vi "MWT NO STIM.vi"() -> ()   [LabVIEW 2015]
uses:
  <vilib>/userdefined/High Color/IMAQdx.ctl
  <vilib>/vision/Image Controls.llb/IMAQ Image.ctl
  <vilib>/DAQmx/write.llb/DAQmx Write (Digital Bool 1Line 1Point).vi
  <vilib>/Utility/config.llb/Read Key (String).vi
  <vilib>/DAQmx/create/channels.llb/DAQmx Create Channel (DO-Digital Output).vi
  <vilib>/DAQmx/miscellaneous.llb/DAQmx Fill In Error Info.vi
  MWT.dll
  <vilib>/vision/driver/NI_Vision_Acquisition_Software.lvlib
  <vilib>/Utility/config.llb/NI_LVConfig.lvlib
panel:
  out "Go":bool
  in  "Turn on external triggering of camera":bool
  in  "User interface display slector":u16(ring)=2 items=["Raw Image", "Memory Image", "Fixed Image", "Nothing"]
  out "Auto-end in (s)":dbl
  out "error out 2":errorcluster
  in  "Minimum time between events(ms)":u32=2000
  in  "custom 1 timing array":dbl[](array[numeric])=[0.0]
  in  "puff timing array":dbl[](array[numeric])=[0.0]
  in  "tap timing array":dbl[](array[numeric])=[0.0]
  in  "custom 2 timing array":dbl[](array[numeric])=[0.0]
  in  "Tap Train Number":i32[][](array[numeric])=[[0, 1]]
  in  "Turn on Background division algorithm":bool
  in  "custom 2 fraction of time between is active":sgl[][](array[numeric])=[[0.0, 0.5]]
  in  "time between custom 2 onset":i32[][](array[numeric])=[[0, 50]]
  in  "custom 1 fraction of time between is active":sgl[][](array[numeric])=[[0.0, 0.5]]
  in  "time between custom 1 onset":i32[][](array[numeric])=[[0, 50]]
  in  "time between puff onset":i32[][](array[numeric])=[[0, 50]]
  in  "puff fraction of time between is active":sgl[][](array[numeric])=[[0.0, 0.5]]
  in  "time between tap onset":i32[][](array[numeric])=[[0, 10]]
  in  "tap fraction of time between is active":sgl[][](array[numeric])=[[0.0, 0.6]]
  in  "Turn on output aggregation?":bool=TRUE
  out "# Custom 2's Delivered":i32
  out "Time until Next Custom 2":dbl
  in  "Custom 2 Signal-high lead up":i32=20
  in  "Custom 2 Signal-high duration":i32=50
  in  "Advanced Custom 2 Settings":bool
  in  "Custom 2 Stimulus Method":u16(ring) items=["Fixed Interval"=0, "Exponential Interval"=2, "Custom"=5]
  in  "Custom 2 Number":i32 caption="# of Puff events"
  in  "Custom 2 Interval":dbl caption="Custom Interval (s)"
  in  "Custom 2 Delay":dbl caption="Puff Onset Delay (s)" format="%#_4g"
  in  "Custom 2":bool
  out "Image Data Input Source":T1(ring)
  in  "Number of Image Adaptation Bands":i32=10
  out "error out":errorcluster
  in  "AVI path":path
  out "Auto-start in (s)":dbl
  in  "Auto-start delay (s)":i32
  in  "Raw Image Save Interval (s)":dbl
  in  "IMAQdx camera interface name":T2="cam0"
  out "Query for Interface?":bool=TRUE
  out "last acquired buffer":i32
  in  "Advanced Settings":bool
  out "# Custom 1's Delivered":i32
  out "Time until Next Custom 1":dbl caption="No Custom 1s"
  in  "Custom 1 Signal-high lead up":i32=20
  in  "Custom 1 Signal-high duration":i32=50
  out "Tracker Handle":i32=1
  out "IMAQ Session":refnum<k11>
  in  "Advanced Custom 1 Settings":bool
  in  "Custom 1 Stimulus Method":u16(ring) items=["Fixed Interval"=0, "Exponential Interval"=2, "Custom"=5]
  in  "Custom 1 Number":i32 caption="# of Puff events"
  in  "Custom 1 Interval":dbl caption="Custom Interval (s)"
  in  "Custom 1 Delay":dbl caption="Puff Onset Delay (s)" format="%#_4g"
  in  "Custom 1":bool
  in  "Image Binning":u16(ring)=1 items=["1"=1, "2"=2, "3"=3, "4"=4]
  in  "Contour?":bool
  in  "AFG resource name":refnum<k15>="COM1"
  out "Proccessing loop stopped?":bool
  in  "Object Border":i32=20
  out "AFG Settings":dbl[][](array[numeric])=[[0.0, 10.0, 1.0]]
  out "AFG instrument handle":refnum<k15> caption="instrument handle out"
  in  "Puff Signal-high lead up":i32=20
  in  "Puff Signal-high duration":i32=50
  in  "Frames of Adaptation":i32=10
  out "# Taps Delivered":i32
  out "# Puffs Delivered":i32
  in  "Skeletonize?":bool
  out "ROI Array":dbl[][](array[numeric])=[[0.0, 0.0, 2350.0, 1726.0, 0.0, 0.0]]
  out "Time until Next Puff":dbl caption="No Puffs"
  out "Seconds into Experiment":dbl
  out "Objects Found":i32
  in  "Bit Depth from Camera?":bool=TRUE
  in  "Image Bit Depth":u32=8
  in  "Advanced Puff Settings":bool
  in  "Graph Input 4":u16(ring)=9 items=["# objects", "# objects persisting", "Persistence", "Speed", "Angular Speed", "Length", "Relative Length", "Width", "Relative Width", "Aspect", "Relative Aspect", "Head Or Tail Angle", "Pixel Count"]
  in  "Graph Input 3":u16(ring)=3 items=["# objects", "# objects persisting", "Persistence", "Speed", "Angular Speed", "Length", "Relative Length", "Width", "Relative Width", "Aspect", "Relative Aspect", "Head Or Tail Angle", "Pixel Count"]
  in  "Graph Input 2":u16(ring)=1 items=["# objects", "# objects persisting", "Persistence", "Speed", "Angular Speed", "Length", "Relative Length", "Width", "Relative Width", "Aspect", "Relative Aspect", "Head Or Tail Angle", "Pixel Count"]
  in  "Graph Input":u16(ring) items=["# objects", "# objects persisting", "Persistence", "Speed", "Angular Speed", "Length", "Relative Length", "Width", "Relative Width", "Aspect", "Relative Aspect", "Head or Tail Angle", "Pixel Count"]
  out "XY Graph 4":cluster{sgl, sgl}[](graph)
  out "XY Graph 3":cluster{sgl, sgl}[](graph)
  out "XY Graph 2":cluster{sgl, sgl}[](graph)
  out "XY Graph":cluster{sgl, sgl}[](graph)
  out "Time until Next Tap":dbl caption="No Taps"
  in  "Puff Stimulus Method":u16(ring) items=["Fixed Interval"=0, "Exponential Interval"=2, "Custom"=5]
  in  "Tap Pulse Active downtime":i32=120
  in  "Tap Pulse Active duration":i32=120
  in  "Tap Signal-high duration":i32=100
  in  "Tap Signal-high lead up":i32=20
  out "seconds per frame":sgl
  out "error count":i32
  out "First-call":bool=TRUE
  in  "Run":bool
  in  "Adaptation Rate":i32=5 step=1
  out "Directory Exists?":bool
  in  "IMAQ Camera Interface Name":string="img0"
  in  "Display/Don't Display":bool=TRUE
  in  "What to display":u16(ring)=2 items=["Raw Image", "Memory Image", "Fixed Image"]
  out "Image":T3(plugin-control)
  in  "Stop":bool=TRUE
  in  "Set New Reference Object":bool
  in  "Clear Reference Object(s)":bool
  in  "Set Region of Interest":bool
  in  "Clear Region of Interest":bool
  in  "Load":bool
  in  "Save":bool
  in  "Advanced Tap Settings":bool
  in  "Tap Stimulus Method":u16(ring) items=["Fixed Interval"=0, "Exponential Interval"=2, "Custom"=5]
  in  "Puff Number":i32 caption="# of Puff events"
  in  "Puff Interval":dbl caption="Puff Interval (s)"
  in  "Puff Delay":dbl caption="Puff Onset Delay (s)"
  in  "Tap Number":i32 caption="# of Tap events" step=1
  in  "Tap Interval":dbl caption="Tap Interval (s)"
  in  "Tap Delay":dbl caption="Tap Onset Delay (s)"
  in  "Puff":bool
  in  "Tap":bool
  in  "Experiment Duration (s)":dbl
  in  "Prefix":string
  in  "Path":path
  in  "Object Size hysteresis (%)":dbl=10.0 min=0.0001 max=100.0
  in  "Minimum Object Size (pixels)":i32=50
  in  "Maximum Object Size (pixels)":i32=6000
  in  "Fill Hysteresis (%)":dbl=50.0 min=0.0001 max=1000.0
  in  "Object Contrast (%)":dbl=10.0 min=0.0001 max=100.0
  in  "Type of object to track":bool
  # "Display"
  # "Do not display"
  # "Multi-Worm Tracker\n(Release -)\n(Without Stimulus)"
  # "Region of Interest"
  # "Reference Object"
  # "Display"
  # "Object Tracker Settings"
  # "Contrast"
  # "Size"
  # "Bright Objects"
  # "Dark Objects"
  # "Data Ouput Settings"
  # "Stimulus Settings"
  # "On"
  # "On"
  # "On"
  # "On"
  # "Off"
  # "Off"
  # "Off"
  # "Off"
  # "Onset delay (s)"
  # "Interval (s)"
  # "Events (#)"
  # "Configuration"
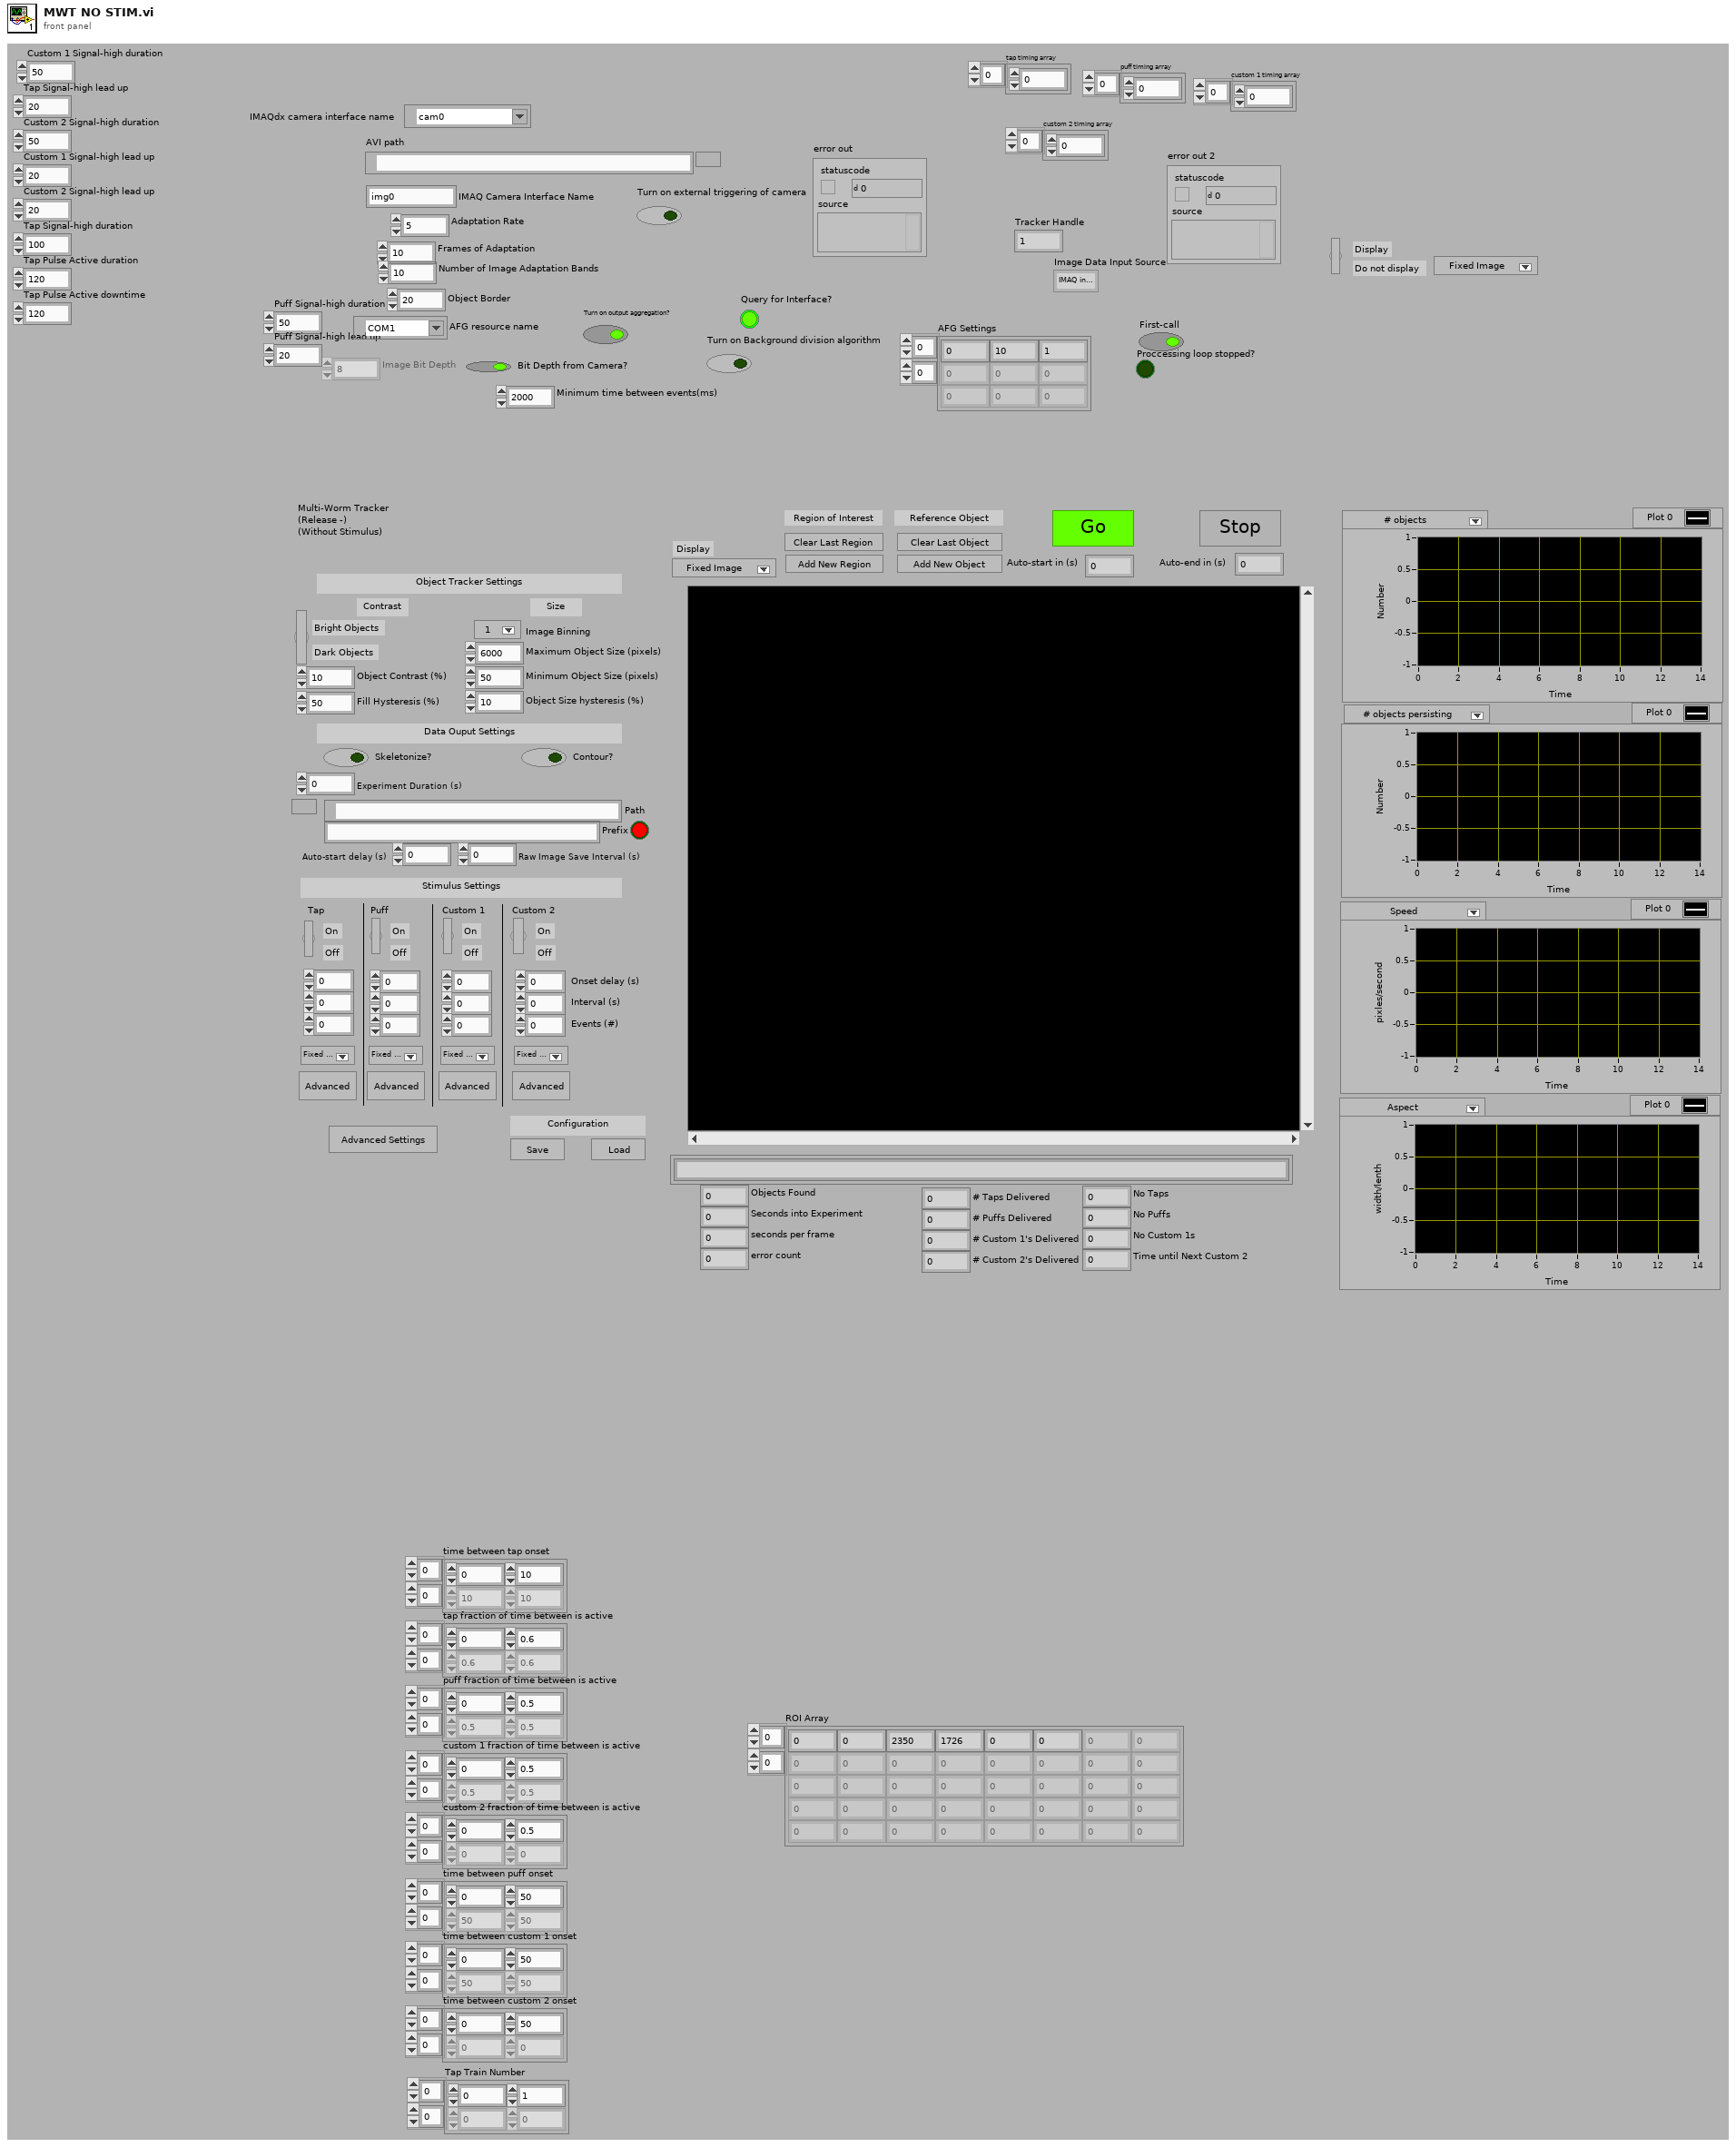
[diagram p1: front panel]
types:
  T1 = enum32{"IMAQ interface", "IMAQdx interface", "AVI file"}
  T2 = typedef "IMAQdx.ctl" = refnum<k21>
  T3 = typedef "IMAQ Image.ctl" = refnum<image>
  T4 = cluster{"Puff":refnum<vi>, "Puff Delay":refnum<vi>, "Puff Interval":refnum<vi>, "Puff Number":refnum<vi>, "Puff Stimulus Method":refnum<vi>}
  T5 = cluster{"Custom 2":refnum<vi>, "Custom 2 Delay":refnum<vi>, "Custom 2 Interval":refnum<vi>, "Custom 2 Number":refnum<vi>, "Custom 2 Stimulus Method":refnum<vi>}
  T6 = cluster{"Custom 1":refnum<vi>, "Custom 1 Delay":refnum<vi>, "Custom 1 Interval":refnum<vi>, "Custom 1 Number":refnum<vi>, "Custom 1 Stimulus Method":refnum<vi>}
  T7 = cluster{"Tap":refnum<vi>, "Tap Delay":refnum<vi>, "Tap Interval":refnum<vi>, "Tap Number":refnum<vi>, "Tap Stimulus Method":refnum<vi>}
  T8 = cluster{cluster{"Tap":refnum<vi>, "Tap Delay":refnum<vi>, "Tap Interval":refnum<vi>, "Tap Number":refnum<vi>, "Tap Stimulus Method":refnum<vi>}, cluster{"Puff":refnum<vi>, "Puff Delay":refnum<vi>, "Puff Interval":refnum<vi>, "Puff Number":refnum<vi>, "Puff Stimulus Method":refnum<vi>}, cluster{"Custom 1":refnum<vi>, "Custom 1 Delay":refnum<vi>, "Custom 1 Interval":refnum<vi>, "Custom 1 Number":refnum<vi>, "Custom 1 Stimulus Method":refnum<vi>}, cluster{"Custom 2":refnum<vi>, "Custom 2 Delay":refnum<vi>, "Custom 2 Interval":refnum<vi>, "Custom 2 Number":refnum<vi>, "Custom 2 Stimulus Method":refnum<vi>}}
  T9 = cluster{"Run":refnum<vi>, "Set Region of Interest":refnum<vi>, "Clear Region of Interest":refnum<vi>, "Clear Reference Object(s)":refnum<vi>, "Set New Reference Object":refnum<vi>, "Advanced Settings":refnum<vi>}
  T10 = cluster{"Path":refnum<vi>, "Prefix":refnum<vi>, "Type of object to track":refnum<vi>, "Object Contrast (%)":refnum<vi>, "Fill Hysteresis (%)":refnum<vi>, "Maximum Object Size (pixels)":refnum<vi>, "Minimum Object Size (pixels)":refnum<vi>, "Object Size hysteresis (%)":refnum<vi>, "Image Binning":refnum<vi>, "Contour?":refnum<vi>, "Skeletonize?":refnum<vi>, "Frames of Adaptation":refnum<vi>, "Adaptation Rate":refnum<vi>, "Object Border":refnum<vi>, "Image Bit Depth":refnum<vi>, "Bit Depth from Camera?":refnum<vi>, "AFG resource name":refnum<vi>, "IMAQ Camera Interface Name":refnum<vi>, "Auto-start delay (s)":refnum<vi>, "Number of Image Adaptation Bands":refnum<vi>, "Experiment Duration (s)":refnum<vi>, "Tap":refnum<vi>, "Tap Delay":refnum<vi>, "Tap Interval":refnum<vi>, "Tap Number":refnum<vi>, "Tap Stimulus Method":refnum<vi>, "Advanced Tap Settings":refnum<vi>, "Puff":refnum<vi>, "Puff Delay":refnum<vi>, "Puff Interval":refnum<vi>, "Puff Number":refnum<vi>, "Puff Stimulus Method":refnum<vi>, "Advanced Puff Settings":refnum<vi>, "Custom 1":refnum<vi>, "Custom 1 Delay":refnum<vi>, "Custom 1 Interval":refnum<vi>, "Custom 1 Number":refnum<vi>, "Custom 1 Stimulus Method":refnum<vi>, "Advanced Custom 1 Settings":refnum<vi>, "puff fraction of time between is active":refnum<vi>, "time between puff onset":refnum<vi>, "tap fraction of time between is active":refnum<vi>, "time between tap onset":refnum<vi>, "Tap Train Number":refnum<vi>, "custom 1 fraction of time between is active":refnum<vi>, "time between custom 1 onset":refnum<vi>, "Custom 2":refnum<vi>, "Custom 2 Delay":refnum<vi>, "Custom 2 Interval":refnum<vi>, "Custom 2 Number":refnum<vi>, "Custom 2 Stimulus Method":refnum<vi>, "Advanced Custom 2 Settings":refnum<vi>, "custom 2 fraction of time between is active":refnum<vi>, "time between custom 2 onset":refnum<vi>, "Save":refnum<vi>, "Load":refnum<vi>, "Raw Image Save Interval (s)":refnum<vi>, "Turn on output aggregation?":refnum<vi>, "Turn on Background division algorithm":refnum<vi>, "Turn on external triggering of camera":refnum<vi>}
  T11 = cluster{cluster{cluster{"Tap":refnum<vi>, "Tap Delay":refnum<vi>, "Tap Interval":refnum<vi>, "Tap Number":refnum<vi>, "Tap Stimulus Method":refnum<vi>}, cluster{"Puff":refnum<vi>, "Puff Delay":refnum<vi>, "Puff Interval":refnum<vi>, "Puff Number":refnum<vi>, "Puff Stimulus Method":refnum<vi>}, cluster{"Custom 1":refnum<vi>, "Custom 1 Delay":refnum<vi>, "Custom 1 Interval":refnum<vi>, "Custom 1 Number":refnum<vi>, "Custom 1 Stimulus Method":refnum<vi>}, cluster{"Custom 2":refnum<vi>, "Custom 2 Delay":refnum<vi>, "Custom 2 Interval":refnum<vi>, "Custom 2 Number":refnum<vi>, "Custom 2 Stimulus Method":refnum<vi>}}, cluster{"Path":refnum<vi>, "Prefix":refnum<vi>, "Type of object to track":refnum<vi>, "Object Contrast (%)":refnum<vi>, "Fill Hysteresis (%)":refnum<vi>, "Maximum Object Size (pixels)":refnum<vi>, "Minimum Object Size (pixels)":refnum<vi>, "Object Size hysteresis (%)":refnum<vi>, "Image Binning":refnum<vi>, "Contour?":refnum<vi>, "Skeletonize?":refnum<vi>, "Frames of Adaptation":refnum<vi>, "Adaptation Rate":refnum<vi>, "Object Border":refnum<vi>, "Image Bit Depth":refnum<vi>, "Bit Depth from Camera?":refnum<vi>, "AFG resource name":refnum<vi>, "IMAQ Camera Interface Name":refnum<vi>, "Auto-start delay (s)":refnum<vi>, "Number of Image Adaptation Bands":refnum<vi>, "Experiment Duration (s)":refnum<vi>, "Tap":refnum<vi>, "Tap Delay":refnum<vi>, "Tap Interval":refnum<vi>, "Tap Number":refnum<vi>, "Tap Stimulus Method":refnum<vi>, "Advanced Tap Settings":refnum<vi>, "Puff":refnum<vi>, "Puff Delay":refnum<vi>, "Puff Interval":refnum<vi>, "Puff Number":refnum<vi>, "Puff Stimulus Method":refnum<vi>, "Advanced Puff Settings":refnum<vi>, "Custom 1":refnum<vi>, "Custom 1 Delay":refnum<vi>, "Custom 1 Interval":refnum<vi>, "Custom 1 Number":refnum<vi>, "Custom 1 Stimulus Method":refnum<vi>, "Advanced Custom 1 Settings":refnum<vi>, "puff fraction of time between is active":refnum<vi>, "time between puff onset":refnum<vi>, "tap fraction of time between is active":refnum<vi>, "time between tap onset":refnum<vi>, "Tap Train Number":refnum<vi>, "custom 1 fraction of time between is active":refnum<vi>, "time between custom 1 onset":refnum<vi>, "Custom 2":refnum<vi>, "Custom 2 Delay":refnum<vi>, "Custom 2 Interval":refnum<vi>, "Custom 2 Number":refnum<vi>, "Custom 2 Stimulus Method":refnum<vi>, "Advanced Custom 2 Settings":refnum<vi>, "custom 2 fraction of time between is active":refnum<vi>, "time between custom 2 onset":refnum<vi>, "Save":refnum<vi>, "Load":refnum<vi>, "Raw Image Save Interval (s)":refnum<vi>, "Turn on output aggregation?":refnum<vi>, "Turn on Background division algorithm":refnum<vi>, "Turn on external triggering of camera":refnum<vi>}, cluster{"Run":refnum<vi>, "Set Region of Interest":refnum<vi>, "Clear Region of Interest":refnum<vi>, "Clear Reference Object(s)":refnum<vi>, "Set New Reference Object":refnum<vi>, "Advanced Settings":refnum<vi>}}
  T12 = cluster{"Value":bool, "Value":dbl, "Value":dbl, "Value":i32, "Value":u16}
  T13 = typedef "AviRefnum.ctl" = refnum<k1>
  T14 = cluster{"IMAQ Session Out":refnum<k11>, "Avi Refnum":T13, "Value":enum32{"IMAQ interface", "IMAQdx interface", "AVI file"}, "Session Out":T2, "Value":bool}
  T15 = cluster{"Value":refnum<k11>, "Value":refnum<k1>, "Value":enum32{"IMAQ interface", "IMAQdx interface", "AVI file"}, cluster{"Value":string, "Value":T2, "Value":path}, bool, "Value":bool}
  T16 = cluster{"Value":string, "Value":T2, "Value":path}
  T17 = cluster{"Value":refnum<k11>, "Value":refnum<k1>, "Value":enum32{"IMAQ interface", "IMAQdx interface", "AVI file"}}
  T18 = cluster{"Value":refnum<k11>, "Value":refnum<k1>, "Value":enum32{"IMAQ interface", "IMAQdx interface", "AVI file"}, "Value":T2, "Value":bool}
  T19 = typedef "Image Type" = u32
  T20 = cluster{"Value":path, "Value":string, "Value":bool, "Value":dbl, "Value":dbl, "Value":i32, "Value":i32, "Value":dbl, "Value":u16, "Value":bool, "Value":bool, "Value":i32, "Value":i32, "Value":i32, "Value":u32, "Value":i32, "Value":bool}
  T21 = cluster{"AFG Settings":dbl[][], "tap timing array":dbl[], "puff timing array":dbl[], "custom timing array":dbl[], "custom 2 timing array":dbl[], cluster{cluster{"Tap":refnum<vi>, "Tap Delay":refnum<vi>, "Tap Interval":refnum<vi>, "Tap Number":refnum<vi>, "Tap Stimulus Method":refnum<vi>}, cluster{"Puff":refnum<vi>, "Puff Delay":refnum<vi>, "Puff Interval":refnum<vi>, "Puff Number":refnum<vi>, "Puff Stimulus Method":refnum<vi>}, cluster{"Custom 1":refnum<vi>, "Custom 1 Delay":refnum<vi>, "Custom 1 Interval":refnum<vi>, "Custom 1 Number":refnum<vi>, "Custom 1 Stimulus Method":refnum<vi>}, cluster{"Custom 2":refnum<vi>, "Custom 2 Delay":refnum<vi>, "Custom 2 Interval":refnum<vi>, "Custom 2 Number":refnum<vi>, "Custom 2 Stimulus Method":refnum<vi>}}, cluster{"Path":refnum<vi>, "Prefix":refnum<vi>, "Type of object to track":refnum<vi>, "Object Contrast (%)":refnum<vi>, "Fill Hysteresis (%)":refnum<vi>, "Maximum Object Size (pixels)":refnum<vi>, "Minimum Object Size (pixels)":refnum<vi>, "Object Size hysteresis (%)":refnum<vi>, "Image Binning":refnum<vi>, "Contour?":refnum<vi>, "Skeletonize?":refnum<vi>, "Frames of Adaptation":refnum<vi>, "Adaptation Rate":refnum<vi>, "Object Border":refnum<vi>, "Image Bit Depth":refnum<vi>, "Bit Depth from Camera?":refnum<vi>, "AFG resource name":refnum<vi>, "IMAQ Camera Interface Name":refnum<vi>, "Auto-start delay (s)":refnum<vi>, "Number of Image Adaptation Bands":refnum<vi>, "Experiment Duration (s)":refnum<vi>, "Tap":refnum<vi>, "Tap Delay":refnum<vi>, "Tap Interval":refnum<vi>, "Tap Number":refnum<vi>, "Tap Stimulus Method":refnum<vi>, "Advanced Tap Settings":refnum<vi>, "Puff":refnum<vi>, "Puff Delay":refnum<vi>, "Puff Interval":refnum<vi>, "Puff Number":refnum<vi>, "Puff Stimulus Method":refnum<vi>, "Advanced Puff Settings":refnum<vi>, "Custom 1":refnum<vi>, "Custom 1 Delay":refnum<vi>, "Custom 1 Interval":refnum<vi>, "Custom 1 Number":refnum<vi>, "Custom 1 Stimulus Method":refnum<vi>, "Advanced Custom 1 Settings":refnum<vi>, "puff fraction of time between is active":refnum<vi>, "time between puff onset":refnum<vi>, "tap fraction of time between is active":refnum<vi>, "time between tap onset":refnum<vi>, "Tap Train Number":refnum<vi>, "custom 1 fraction of time between is active":refnum<vi>, "time between custom 1 onset":refnum<vi>, "Custom 2":refnum<vi>, "Custom 2 Delay":refnum<vi>, "Custom 2 Interval":refnum<vi>, "Custom 2 Number":refnum<vi>, "Custom 2 Stimulus Method":refnum<vi>, "Advanced Custom 2 Settings":refnum<vi>, "custom 2 fraction of time between is active":refnum<vi>, "time between custom 2 onset":refnum<vi>, "Save":refnum<vi>, "Load":refnum<vi>, "Raw Image Save Interval (s)":refnum<vi>, "Turn on output aggregation?":refnum<vi>, "Turn on Background division algorithm":refnum<vi>, "Turn on external triggering of camera":refnum<vi>}, "output values cluster":cluster{"Value":bool, "Value":dbl, "Value":dbl, "Value":dbl, "Value":u16}, "output values cluster":cluster{"Value":bool, "Value":dbl, "Value":dbl, "Value":dbl, "Value":u16}, "output values cluster":cluster{"Value":bool, "Value":dbl, "Value":dbl, "Value":dbl, "Value":u16}, "output values cluster":cluster{"Value":bool, "Value":dbl, "Value":dbl, "Value":dbl, "Value":u16}}
  T22 = cluster{cluster{"Value":refnum<k11>, "Avi Refnum":T13, "Value":enum32{"IMAQ interface", "IMAQdx interface", "AVI file"}, "Value":T2, "Value":bool}, "Value":i32, "Value":i32}
  T23 = cluster{"output values cluster":cluster{"Value":bool, "Value":dbl, "Value":dbl, "Value":dbl, "Value":u16}, "Output Array":dbl[], "output values cluster":cluster{"Value":bool, "Value":dbl, "Value":dbl, "Value":dbl, "Value":u16}, "Output Array":dbl[], "output values cluster":cluster{"Value":bool, "Value":dbl, "Value":dbl, "Value":dbl, "Value":u16}, "Output Array":dbl[], "AFG Settings":dbl[][], "output values cluster":cluster{"Value":bool, "Value":dbl, "Value":dbl, "Value":dbl, "Value":u16}, "Output Array":dbl[]}
  T24 = cluster{cluster{cluster{"Value":refnum<k11>, "Avi Refnum":T13, "Value":enum32{"IMAQ interface", "IMAQdx interface", "AVI file"}, "Value":T2, "Value":bool}, "Value":i32, "Value":i32}, cluster{"Run":refnum<vi>, "Set Region of Interest":refnum<vi>, "Clear Region of Interest":refnum<vi>, "Clear Reference Object(s)":refnum<vi>, "Set New Reference Object":refnum<vi>, "Advanced Settings":refnum<vi>}, "Image Bit Depth":u32}
  T25 = cluster{"Value":bool, "Value":dbl, "Value":dbl, "Value":dbl, "Value":u16}
  T26 = cluster{cluster{cluster{"Value":refnum<k11>, "Avi Refnum":T13, "Value":enum32{"IMAQ interface", "IMAQdx interface", "AVI file"}, "Value":T2, "Value":bool}, "Value":i32, "Value":i32}, cluster{"Path":refnum<vi>, "Prefix":refnum<vi>, "Type of object to track":refnum<vi>, "Object Contrast (%)":refnum<vi>, "Fill Hysteresis (%)":refnum<vi>, "Maximum Object Size (pixels)":refnum<vi>, "Minimum Object Size (pixels)":refnum<vi>, "Object Size hysteresis (%)":refnum<vi>, "Image Binning":refnum<vi>, "Contour?":refnum<vi>, "Skeletonize?":refnum<vi>, "Frames of Adaptation":refnum<vi>, "Adaptation Rate":refnum<vi>, "Object Border":refnum<vi>, "Image Bit Depth":refnum<vi>, "Bit Depth from Camera?":refnum<vi>, "AFG resource name":refnum<vi>, "IMAQ Camera Interface Name":refnum<vi>, "Auto-start delay (s)":refnum<vi>, "Number of Image Adaptation Bands":refnum<vi>, "Experiment Duration (s)":refnum<vi>, "Tap":refnum<vi>, "Tap Delay":refnum<vi>, "Tap Interval":refnum<vi>, "Tap Number":refnum<vi>, "Tap Stimulus Method":refnum<vi>, "Advanced Tap Settings":refnum<vi>, "Puff":refnum<vi>, "Puff Delay":refnum<vi>, "Puff Interval":refnum<vi>, "Puff Number":refnum<vi>, "Puff Stimulus Method":refnum<vi>, "Advanced Puff Settings":refnum<vi>, "Custom 1":refnum<vi>, "Custom 1 Delay":refnum<vi>, "Custom 1 Interval":refnum<vi>, "Custom 1 Number":refnum<vi>, "Custom 1 Stimulus Method":refnum<vi>, "Advanced Custom 1 Settings":refnum<vi>, "puff fraction of time between is active":refnum<vi>, "time between puff onset":refnum<vi>, "tap fraction of time between is active":refnum<vi>, "time between tap onset":refnum<vi>, "Tap Train Number":refnum<vi>, "custom 1 fraction of time between is active":refnum<vi>, "time between custom 1 onset":refnum<vi>, "Custom 2":refnum<vi>, "Custom 2 Delay":refnum<vi>, "Custom 2 Interval":refnum<vi>, "Custom 2 Number":refnum<vi>, "Custom 2 Stimulus Method":refnum<vi>, "Advanced Custom 2 Settings":refnum<vi>, "custom 2 fraction of time between is active":refnum<vi>, "time between custom 2 onset":refnum<vi>, "Save":refnum<vi>, "Load":refnum<vi>, "Raw Image Save Interval (s)":refnum<vi>, "Turn on output aggregation?":refnum<vi>, "Turn on Background division algorithm":refnum<vi>, "Turn on external triggering of camera":refnum<vi>}, "ROI Array":dbl[][], "settings value cluster":cluster{"Value":path, "Value":string, "Value":bool, "Value":dbl, "Value":dbl, "Value":i32, "Value":i32, "Value":dbl, "Value":u16, "Value":bool, "Value":bool, "Value":i32, "Value":i32, "Value":i32, "Value":u32, "Value":i32, "Value":bool}, "AFG Settings":dbl[][], "Output Array":dbl[], "Output Array":dbl[], "Output Array":dbl[], "Output Array":dbl[]}
  T27 = cluster{"Output  ROI Array":dbl[][], "settings value cluster":cluster{"Value":path, "Value":string, "Value":bool, "Value":dbl, "Value":dbl, "Value":i32, "Value":i32, "Value":dbl, "Value":u16, "Value":bool, "Value":bool, "Value":i32, "Value":i32, "Value":i32, "Value":u32, "Value":i32, "Value":bool}, "AFG Settings":dbl[][], "tap timing array":dbl[], "puff timing array":dbl[], "custom timing array":dbl[], "custom 2 timing array":dbl[]}
  T28 = cluster{cluster{"Path":refnum<vi>, "Prefix":refnum<vi>, "Type of object to track":refnum<vi>, "Object Contrast (%)":refnum<vi>, "Fill Hysteresis (%)":refnum<vi>, "Maximum Object Size (pixels)":refnum<vi>, "Minimum Object Size (pixels)":refnum<vi>, "Object Size hysteresis (%)":refnum<vi>, "Image Binning":refnum<vi>, "Contour?":refnum<vi>, "Skeletonize?":refnum<vi>, "Frames of Adaptation":refnum<vi>, "Adaptation Rate":refnum<vi>, "Object Border":refnum<vi>, "Image Bit Depth":refnum<vi>, "Bit Depth from Camera?":refnum<vi>, "AFG resource name":refnum<vi>, "IMAQ Camera Interface Name":refnum<vi>, "Auto-start delay (s)":refnum<vi>, "Number of Image Adaptation Bands":refnum<vi>, "Experiment Duration (s)":refnum<vi>, "Tap":refnum<vi>, "Tap Delay":refnum<vi>, "Tap Interval":refnum<vi>, "Tap Number":refnum<vi>, "Tap Stimulus Method":refnum<vi>, "Advanced Tap Settings":refnum<vi>, "Puff":refnum<vi>, "Puff Delay":refnum<vi>, "Puff Interval":refnum<vi>, "Puff Number":refnum<vi>, "Puff Stimulus Method":refnum<vi>, "Advanced Puff Settings":refnum<vi>, "Custom 1":refnum<vi>, "Custom 1 Delay":refnum<vi>, "Custom 1 Interval":refnum<vi>, "Custom 1 Number":refnum<vi>, "Custom 1 Stimulus Method":refnum<vi>, "Advanced Custom 1 Settings":refnum<vi>, "puff fraction of time between is active":refnum<vi>, "time between puff onset":refnum<vi>, "tap fraction of time between is active":refnum<vi>, "time between tap onset":refnum<vi>, "Tap Train Number":refnum<vi>, "custom 1 fraction of time between is active":refnum<vi>, "time between custom 1 onset":refnum<vi>, "Custom 2":refnum<vi>, "Custom 2 Delay":refnum<vi>, "Custom 2 Interval":refnum<vi>, "Custom 2 Number":refnum<vi>, "Custom 2 Stimulus Method":refnum<vi>, "Advanced Custom 2 Settings":refnum<vi>, "custom 2 fraction of time between is active":refnum<vi>, "time between custom 2 onset":refnum<vi>, "Save":refnum<vi>, "Load":refnum<vi>, "Raw Image Save Interval (s)":refnum<vi>, "Turn on output aggregation?":refnum<vi>, "Turn on Background division algorithm":refnum<vi>, "Turn on external triggering of camera":refnum<vi>}, cluster{"Value":refnum<k11>, "Avi Refnum":T13, "Value":enum32{"IMAQ interface", "IMAQdx interface", "AVI file"}, "Value":T2, "Value":bool}}
  T29 = cluster{cluster{cluster{"Value":refnum<k11>, "Avi Refnum":T13, "Value":enum32{"IMAQ interface", "IMAQdx interface", "AVI file"}, "Value":T2, "Value":bool}, "Value":i32, "Value":i32}, "Image Binning":u16, "Value":u16}
  T30 = cluster{"Acquired Buffer Number":i32, "return type":i32, "destination":i16[][]}
  T31 = cluster{cluster{cluster{"Value":refnum<k11>, "Avi Refnum":T13, "Value":enum32{"IMAQ interface", "IMAQdx interface", "AVI file"}, "Value":T2, "Value":bool}, "Value":i32, "Value":i32}, "ROI Array":dbl[][], "Value":bool, cluster{"Path":refnum<vi>, "Prefix":refnum<vi>, "Type of object to track":refnum<vi>, "Object Contrast (%)":refnum<vi>, "Fill Hysteresis (%)":refnum<vi>, "Maximum Object Size (pixels)":refnum<vi>, "Minimum Object Size (pixels)":refnum<vi>, "Object Size hysteresis (%)":refnum<vi>, "Image Binning":refnum<vi>, "Contour?":refnum<vi>, "Skeletonize?":refnum<vi>, "Frames of Adaptation":refnum<vi>, "Adaptation Rate":refnum<vi>, "Object Border":refnum<vi>, "Image Bit Depth":refnum<vi>, "Bit Depth from Camera?":refnum<vi>, "AFG resource name":refnum<vi>, "IMAQ Camera Interface Name":refnum<vi>, "Auto-start delay (s)":refnum<vi>, "Number of Image Adaptation Bands":refnum<vi>, "Experiment Duration (s)":refnum<vi>, "Tap":refnum<vi>, "Tap Delay":refnum<vi>, "Tap Interval":refnum<vi>, "Tap Number":refnum<vi>, "Tap Stimulus Method":refnum<vi>, "Advanced Tap Settings":refnum<vi>, "Puff":refnum<vi>, "Puff Delay":refnum<vi>, "Puff Interval":refnum<vi>, "Puff Number":refnum<vi>, "Puff Stimulus Method":refnum<vi>, "Advanced Puff Settings":refnum<vi>, "Custom 1":refnum<vi>, "Custom 1 Delay":refnum<vi>, "Custom 1 Interval":refnum<vi>, "Custom 1 Number":refnum<vi>, "Custom 1 Stimulus Method":refnum<vi>, "Advanced Custom 1 Settings":refnum<vi>, "puff fraction of time between is active":refnum<vi>, "time between puff onset":refnum<vi>, "tap fraction of time between is active":refnum<vi>, "time between tap onset":refnum<vi>, "Tap Train Number":refnum<vi>, "custom 1 fraction of time between is active":refnum<vi>, "time between custom 1 onset":refnum<vi>, "Custom 2":refnum<vi>, "Custom 2 Delay":refnum<vi>, "Custom 2 Interval":refnum<vi>, "Custom 2 Number":refnum<vi>, "Custom 2 Stimulus Method":refnum<vi>, "Advanced Custom 2 Settings":refnum<vi>, "custom 2 fraction of time between is active":refnum<vi>, "time between custom 2 onset":refnum<vi>, "Save":refnum<vi>, "Load":refnum<vi>, "Raw Image Save Interval (s)":refnum<vi>, "Turn on output aggregation?":refnum<vi>, "Turn on Background division algorithm":refnum<vi>, "Turn on external triggering of camera":refnum<vi>}, cluster{"Run":refnum<vi>, "Set Region of Interest":refnum<vi>, "Clear Region of Interest":refnum<vi>, "Clear Reference Object(s)":refnum<vi>, "Set New Reference Object":refnum<vi>, "Advanced Settings":refnum<vi>}, "Directory Exists?":refnum<vi>}
  T32 = cluster{cluster{"Value":refnum<k11>, "Avi Refnum":T13, "Value":enum32{"IMAQ interface", "IMAQdx interface", "AVI file"}, "Value":T2, "Value":bool}, i32}
  T33 = cluster{"tap timing array":dbl[], "puff timing array":dbl[], "custom timing array":dbl[], "custom 2 timing array":dbl[]}
  T34 = cluster{"width":u32, "height":u32, "framesPerSecond":u32, "compressionFilter":string, "hasData":bool}
  T35 = cluster{cluster{"Value":refnum<k11>, "Avi Refnum":T13, "Value":enum32{"IMAQ interface", "IMAQdx interface", "AVI file"}, "Value":T2, "Value":bool}, "Value":i32}
  T36 = cluster{"Value":refnum<k11>, "Avi Refnum":T13, "Value":enum32{"IMAQ interface", "IMAQdx interface", "AVI file"}, "Value":T2, "Value":bool}
  T37 = cluster{cluster{cluster{"Value":refnum<k11>, "Avi Refnum":T13, "Value":enum32{"IMAQ interface", "IMAQdx interface", "AVI file"}, "Value":T2, "Value":bool}, "Value":i32}, "Value":i32, "Value":i32, "Value":u16, "Image":T3}
  T38 = cluster{cluster{"Value":refnum<k11>, "Avi Refnum":T13, "Value":enum32{"IMAQ interface", "IMAQdx interface", "AVI file"}, "Value":T2, "Value":bool}, "Acquired Buffer Number":u32}
  T39 = cluster{cluster{"Path":refnum<vi>, "Prefix":refnum<vi>, "Type of object to track":refnum<vi>, "Object Contrast (%)":refnum<vi>, "Fill Hysteresis (%)":refnum<vi>, "Maximum Object Size (pixels)":refnum<vi>, "Minimum Object Size (pixels)":refnum<vi>, "Object Size hysteresis (%)":refnum<vi>, "Image Binning":refnum<vi>, "Contour?":refnum<vi>, "Skeletonize?":refnum<vi>, "Frames of Adaptation":refnum<vi>, "Adaptation Rate":refnum<vi>, "Object Border":refnum<vi>, "Image Bit Depth":refnum<vi>, "Bit Depth from Camera?":refnum<vi>, "AFG resource name":refnum<vi>, "IMAQ Camera Interface Name":refnum<vi>, "Auto-start delay (s)":refnum<vi>, "Number of Image Adaptation Bands":refnum<vi>, "Experiment Duration (s)":refnum<vi>, "Tap":refnum<vi>, "Tap Delay":refnum<vi>, "Tap Interval":refnum<vi>, "Tap Number":refnum<vi>, "Tap Stimulus Method":refnum<vi>, "Advanced Tap Settings":refnum<vi>, "Puff":refnum<vi>, "Puff Delay":refnum<vi>, "Puff Interval":refnum<vi>, "Puff Number":refnum<vi>, "Puff Stimulus Method":refnum<vi>, "Advanced Puff Settings":refnum<vi>, "Custom 1":refnum<vi>, "Custom 1 Delay":refnum<vi>, "Custom 1 Interval":refnum<vi>, "Custom 1 Number":refnum<vi>, "Custom 1 Stimulus Method":refnum<vi>, "Advanced Custom 1 Settings":refnum<vi>, "puff fraction of time between is active":refnum<vi>, "time between puff onset":refnum<vi>, "tap fraction of time between is active":refnum<vi>, "time between tap onset":refnum<vi>, "Tap Train Number":refnum<vi>, "custom 1 fraction of time between is active":refnum<vi>, "time between custom 1 onset":refnum<vi>, "Custom 2":refnum<vi>, "Custom 2 Delay":refnum<vi>, "Custom 2 Interval":refnum<vi>, "Custom 2 Number":refnum<vi>, "Custom 2 Stimulus Method":refnum<vi>, "Advanced Custom 2 Settings":refnum<vi>, "custom 2 fraction of time between is active":refnum<vi>, "time between custom 2 onset":refnum<vi>, "Save":refnum<vi>, "Load":refnum<vi>, "Raw Image Save Interval (s)":refnum<vi>, "Turn on output aggregation?":refnum<vi>, "Turn on Background division algorithm":refnum<vi>, "Turn on external triggering of camera":refnum<vi>}, "appended path":path, "ROI Array":dbl[][], "AFG Settings":dbl[][], "tap timing array":dbl[], "puff timing array":dbl[], "custom timing array":dbl[], "custom 2 timing array":dbl[]}
  T40 = cluster{cluster{"Value":refnum<k11>, "Avi Refnum":T13, "Value":enum32{"IMAQ interface", "IMAQdx interface", "AVI file"}, "Value":T2, "Value":bool}, "Acquired Buffer Number":i32}
  T41 = cluster{"Graph Input":refnum<vi>, "Graph Input 2":refnum<vi>, "Graph Input 3":refnum<vi>, "Graph Input 4":refnum<vi>, "XY Graph":refnum<vi>, "XY Graph 2":refnum<vi>, "XY Graph 3":refnum<vi>, "XY Graph 4":refnum<vi>}
  T42 = cluster{"Value":sgl[][], "Value":i32[][], "Value":i32[][]}
  T43 = cluster{cluster{sgl, sgl}[], cluster{sgl, sgl}[], cluster{sgl, sgl}[], cluster{sgl, sgl}[], cluster{sgl, sgl}[], cluster{sgl, sgl}[], cluster{sgl, sgl}[], cluster{sgl, sgl}[], cluster{sgl, sgl}[], cluster{sgl, sgl}[], cluster{sgl, sgl}[], cluster{sgl, sgl}[], cluster{sgl, sgl}[]}
  T44 = cluster{"custom timing array":dbl[], i32, i32, "Value":bool, i32, "stimulus settings":cluster{"outy3":sgl, "outy3":i32}}
  T45 = cluster{"custom 2 timing array":dbl[], i32, i32, "Value":bool, i32, "stimulus settings":cluster{"outy3":sgl, "outy3":i32}}
  T46 = cluster{"puff timing array":dbl[], i32, i32, "Value":bool, i32, "stimulus settings":cluster{"outy3":sgl, "outy3":i32}}
  T47 = cluster{"tap timing array":dbl[], i32, i32, "Value":bool, i32, "stimulus settings":cluster{"outy3":sgl, "outy3":i32, "Value":i32}}
  T48 = cluster{u32, "millisecond timer value":u32, "millisecond timer value":u32, "Value":u32}
  T49 = cluster{cluster{u32, "millisecond timer value":u32, "millisecond timer value":u32, "Value":u32}, "Time until Next Tap":refnum<vi>, cluster{"tap timing array":dbl[], i32, i32, "Value":bool, i32, "stimulus settings":cluster{"outy3":sgl, "outy3":i32, "Value":i32}}}
  T50 = cluster{cluster{u32, "millisecond timer value":u32, "millisecond timer value":u32, "Value":u32}, "Time until Next Puff":refnum<vi>, cluster{"puff timing array":dbl[], i32, i32, "Value":bool, i32, "stimulus settings":cluster{"outy3":sgl, "outy3":i32}}}
  T51 = cluster{cluster{u32, "millisecond timer value":u32, "millisecond timer value":u32, "Value":u32}, "Time until Next Custom 1":refnum<vi>, cluster{"custom timing array":dbl[], i32, i32, "Value":bool, i32, "stimulus settings":cluster{"outy3":sgl, "outy3":i32}}}
  T52 = cluster{cluster{u32, "millisecond timer value":u32, "millisecond timer value":u32, "Value":u32}, "Time until Next Custom 2":refnum<vi>, cluster{"custom 2 timing array":dbl[], i32, i32, "Value":bool, i32, "stimulus settings":cluster{"outy3":sgl, "outy3":i32}}}
  T53 = cluster{"millisecond timer value":u32, "millisecond timer value":u32, i32, sgl, "Data Cluster":cluster{cluster{sgl, sgl}[], cluster{sgl, sgl}[], cluster{sgl, sgl}[], cluster{sgl, sgl}[], cluster{sgl, sgl}[], cluster{sgl, sgl}[], cluster{sgl, sgl}[], cluster{sgl, sgl}[], cluster{sgl, sgl}[], cluster{sgl, sgl}[], cluster{sgl, sgl}[], cluster{sgl, sgl}[], cluster{sgl, sgl}[]}, "Value":i32, cluster{"Graph Input":refnum<vi>, "Graph Input 2":refnum<vi>, "Graph Input 3":refnum<vi>, "Graph Input 4":refnum<vi>, "XY Graph":refnum<vi>, "XY Graph 2":refnum<vi>, "XY Graph 3":refnum<vi>, "XY Graph 4":refnum<vi>}}
  T54 = cluster{i32, "Tap Number":i32, "Elapsed Time":i32}
  T55 = cluster{"Elapsed Time":i32, "Data Cluster":cluster{cluster{sgl, sgl}[], cluster{sgl, sgl}[], cluster{sgl, sgl}[], cluster{sgl, sgl}[], cluster{sgl, sgl}[], cluster{sgl, sgl}[], cluster{sgl, sgl}[], cluster{sgl, sgl}[], cluster{sgl, sgl}[], cluster{sgl, sgl}[], cluster{sgl, sgl}[], cluster{sgl, sgl}[], cluster{sgl, sgl}[]}}
  T56 = cluster{i32, "Value":i32, "Value":u16, sgl, "Value":u16, "Value":bool, "Value":u32, "Image Out":T3, "Image Pixels (I16)":i16[][], i32[]}
  T57 = cluster{"return value":i32, "return value":i32, "Image Pixels (I16) out":i16[][], "coordinates":i32[]}
  T58 = typedef "NI_LVConfig.lvlib/Config Data RefNum.ctl" = refnum<k1>
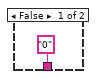
[diagram p2: hidden frame]
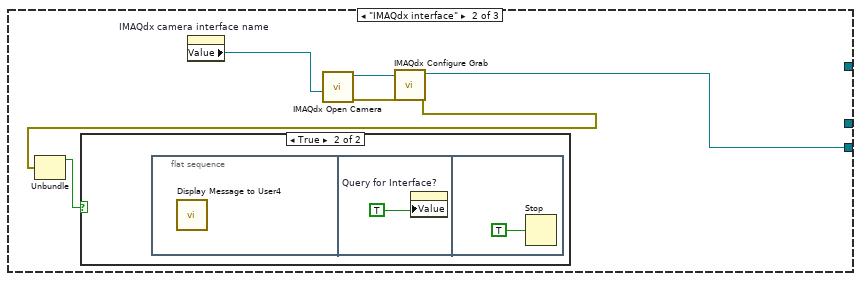
[diagram p5: hidden frame]
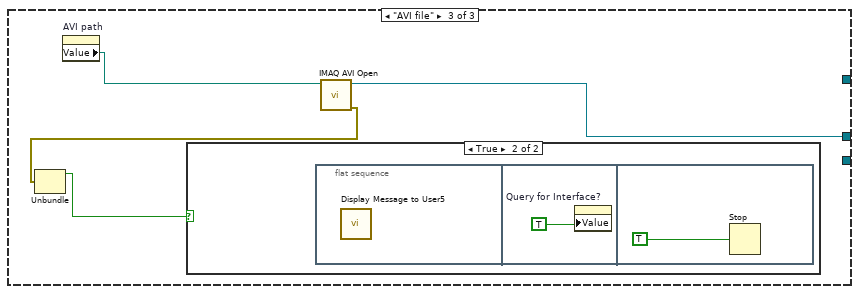
[diagram p7: hidden frame]
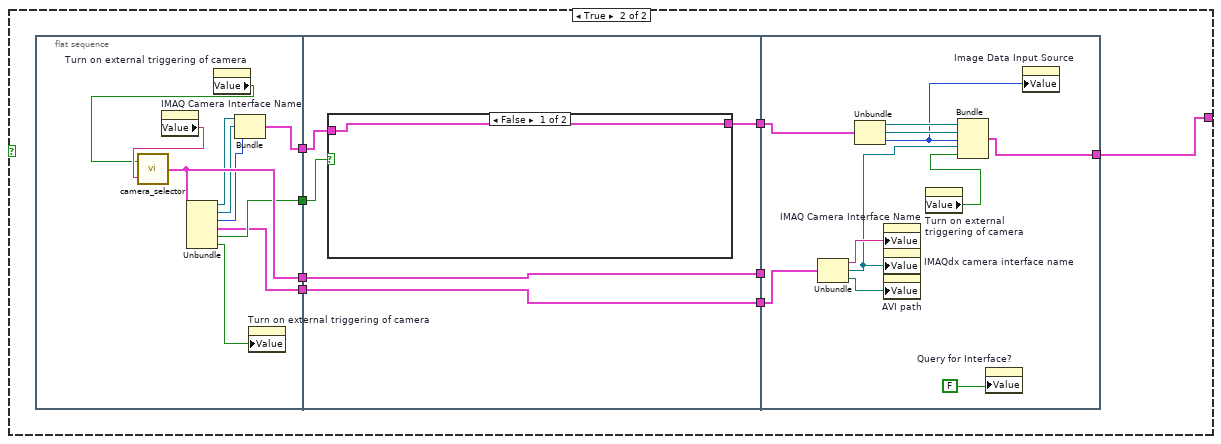
[diagram p9: hidden frame]
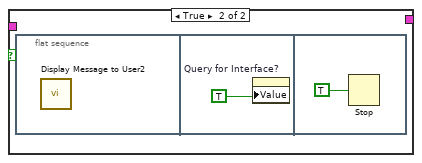
[diagram p10: hidden frame]
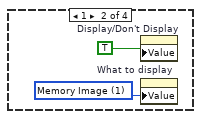
[diagram p16: hidden frame]
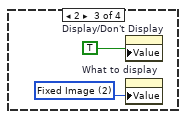
[diagram p17: hidden frame]
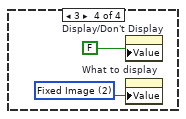
[diagram p18: hidden frame]
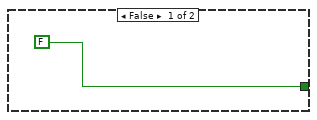
[diagram p19: hidden frame]
diagram:
  w7 = cluster{sgl, sgl}[] [] ("XY Graph")
  w28 = 0
  # "Stimulus counter trigger arrays"
  # "Stimulus event timing arrays"
  # "Copyright (C) 2007 - 2010 Howard Hughes Medical Institute\nCopyright (C) 2007 - 2010 Rex A. Kerr, Nicholas A. Swierczek\n \nThis file is a part of the Multi-Worm Tracker and is distributed under the\nterms of the GNU Lesser General Public Licence version 2.1 (LGPL 2.1).\nFor details, see GPL2.txt and LGPL2.1.txt, or http://www.gnu.org/licences\n \nTo contact the authors, email kerrlab@users.sourceforge.net."
  # "Device Start Timing Control"
  # "Main Controls Cluster"
  # "Assorted buttons for advanced settings/ROI/reference objects"
  # "Stimulus Timing Controls"
  # "Exp. Duration"
  # "Array of ROIs"
  # "Statistics data controls"
  # "Display Controls; \ndisplay type and display on/off toggle"
  # "Settigns-related buttons"
  # "ROI-related buttons"
  # "Reference Object-related buttons"
  # "Overall control buttons"
  # "Image Bit Depth Control"
  # "Function Generator Settings"
  # "Image/Tracking Parameters"
  # "Blob Tracking Parameters"
  # "State variables"
  # "Images"
  # "Hardware System names/handles"
  # "Graph FP objects and controls"
  # "Stimulus delivery control parameters"
  # "Stimulus control signal parameters"
  # "Front panel indicators"
  # "Data output parameters"
  # "References to the front panel controls"
  n1 = control-ref of="AFG resource name"() -> (w74:refnum<vi>)
  n2 = control-ref of="Turn on Background division algorithm"() -> (w8:refnum<vi>)
  n3 = control-ref of="Turn on external triggering of camera"() -> (w6:refnum<vi>)
  n4 = control-ref of="Turn on output aggregation?"() -> (w9:refnum<vi>)
  n5 = control-ref of="Run"() -> (w105:refnum<vi>)
  n6 = control-ref of="Save"() -> (w20:refnum<vi>)
  n7 = control-ref of="Load"() -> (w21:refnum<vi>)
  n8 = control-ref of="Set Region of Interest"() -> (w119:refnum<vi>)
  n9 = control-ref of="Clear Region of Interest"() -> (w122:refnum<vi>)
  n10 = control-ref of="Clear Reference Object(s)"() -> (w121:refnum<vi>)
  n11 = control-ref of="Set New Reference Object"() -> (w120:refnum<vi>)
  n12 = control-ref of="Advanced Settings"() -> (w91:refnum<vi>)
  n13 = control-ref of="Custom 2"() -> (w12:refnum<vi>)
  n14 = control-ref of="Advanced Custom 2 Settings"() -> (w17:refnum<vi>)
  n15 = control-ref of="Tap"() -> (w53:refnum<vi>)
  n16 = control-ref of="Advanced Tap Settings"() -> (w48:refnum<vi>)
  n17 = control-ref of="Puff"() -> (w47:refnum<vi>)
  n18 = control-ref of="Advanced Puff Settings"() -> (w42:refnum<vi>)
  n19 = control-ref of="Custom 1"() -> (w41:refnum<vi>)
  n20 = control-ref of="Advanced Custom 1 Settings"() -> (w36:refnum<vi>)
  n21 = control-ref of="Type of object to track"() -> (w88:refnum<vi>)
  n22 = control-ref of="Contour?"() -> (w81:refnum<vi>)
  n23 = control-ref of="Skeletonize?"() -> (w80:refnum<vi>)
  n24 = control-ref of="Bit Depth from Camera?"() -> (w75:refnum<vi>)
  n25 = control-ref of="Raw Image Save Interval (s)"() -> (w11:refnum<vi>)
  n26 = control-ref of="Custom 2"() -> (w23:refnum<vi>)
  n27 = control-ref of="Custom 2 Delay"() -> (w13:refnum<vi>)
  n28 = control-ref of="Custom 2 Interval"() -> (w14:refnum<vi>)
  n29 = control-ref of="Custom 2 Number"() -> (w15:refnum<vi>)
  n30 = control-ref of="Custom 1"() -> (w96:refnum<vi>)
  n31 = control-ref of="Auto-start delay (s)"() -> (w56:refnum<vi>)
  n32 = control-ref of="Number of Image Adaptation Bands"() -> (w55:refnum<vi>)
  n33 = control-ref of="Experiment Duration (s)"() -> (w54:refnum<vi>)
  n34 = control-ref of="Tap Delay"() -> (w52:refnum<vi>)
  n35 = control-ref of="Tap Interval"() -> (w51:refnum<vi>)
  n36 = control-ref of="Tap Number"() -> (w50:refnum<vi>)
  n37 = control-ref of="Puff Delay"() -> (w46:refnum<vi>)
  n38 = control-ref of="Puff Interval"() -> (w45:refnum<vi>)
  n39 = control-ref of="Puff Number"() -> (w44:refnum<vi>)
  n40 = control-ref of="Custom 1 Delay"() -> (w40:refnum<vi>)
  n41 = control-ref of="Custom 1 Interval"() -> (w39:refnum<vi>)
  n42 = control-ref of="Custom 1 Number"() -> (w38:refnum<vi>)
  n43 = control-ref of="Object Contrast (%)"() -> (w87:refnum<vi>)
  n44 = control-ref of="Fill Hysteresis (%)"() -> (w86:refnum<vi>)
  n45 = control-ref of="Maximum Object Size (pixels)"() -> (w85:refnum<vi>)
  n46 = control-ref of="Minimum Object Size (pixels)"() -> (w84:refnum<vi>)
  n47 = control-ref of="Object Size hysteresis (%)"() -> (w83:refnum<vi>)
  n48 = control-ref of="Frames of Adaptation"() -> (w79:refnum<vi>)
  n49 = control-ref of="Adaptation Rate"() -> (w78:refnum<vi>)
  n50 = control-ref of="Object Border"() -> (w77:refnum<vi>)
  n51 = control-ref of="Image Bit Depth"() -> (w76:refnum<vi>)
  n52 = control-ref of="Puff"() -> (w113:refnum<vi>)
  n53 = control-ref of="custom 2 fraction of time between is active"() -> (w18:refnum<vi>)
  n54 = control-ref of="time between custom 2 onset"() -> (w19:refnum<vi>)
  n55 = control-ref of="Prefix"() -> (w89:refnum<vi>)
  n56 = control-ref of="IMAQ Camera Interface Name"() -> (w73:refnum<vi>)
  n57 = control-ref of="puff fraction of time between is active"() -> (w35:refnum<vi>)
  n58 = control-ref of="time between puff onset"() -> (w34:refnum<vi>)
  n59 = control-ref of="tap fraction of time between is active"() -> (w33:refnum<vi>)
  n60 = control-ref of="time between tap onset"() -> (w32:refnum<vi>)
  n61 = control-ref of="Tap Train Number"() -> (w31:refnum<vi>)
  n62 = control-ref of="custom 1 fraction of time between is active"() -> (w30:refnum<vi>)
  n63 = control-ref of="time between custom 1 onset"() -> (w29:refnum<vi>)
  n64 = control-ref of="Custom 2 Interval"() -> (w25:refnum<vi>)
  n65 = control-ref of="Custom 2 Number"() -> (w26:refnum<vi>)
  n66 = control-ref of="Custom 1 Interval"() -> (w94:refnum<vi>)
  n67 = control-ref of="Custom 1 Number"() -> (w93:refnum<vi>)
  n68 = control-ref of="Custom 2 Delay"() -> (w24:refnum<vi>)
  n69 = control-ref of="Custom 2 Stimulus Method"() -> (w16:refnum<vi>)
  n70 = control-ref of="Tap"() -> (w117:refnum<vi>)
  n71 = control-ref of="Custom 1 Delay"() -> (w95:refnum<vi>)
  n72 = control-ref of="Path"() -> (w90:refnum<vi>)
  n73 = control-ref of="Tap Stimulus Method"() -> (w49:refnum<vi>)
  n74 = control-ref of="Puff Stimulus Method"() -> (w43:refnum<vi>)
  n75 = control-ref of="Custom 1 Stimulus Method"() -> (w37:refnum<vi>)
  n76 = control-ref of="Image Binning"() -> (w82:refnum<vi>)
  n77 = control-ref of="Puff Delay"() -> (w112:refnum<vi>)
  n78 = control-ref of="Puff Interval"() -> (w111:refnum<vi>)
  n79 = control-ref of="Puff Number"() -> (w110:refnum<vi>)
  n80 = control-ref of="Custom 2 Stimulus Method"() -> (w27:refnum<vi>)
  n81 = control-ref of="Tap Delay"() -> (w116:refnum<vi>)
  n82 = control-ref of="Tap Interval"() -> (w115:refnum<vi>)
  n83 = control-ref of="Tap Number"() -> (w114:refnum<vi>)
  n84 = control-ref of="Custom 1 Stimulus Method"() -> (w92:refnum<vi>)
  n85 = control-ref of="Puff Stimulus Method"() -> (w108:refnum<vi>)
  n86 = control-ref of="Tap Stimulus Method"() -> (w109:refnum<vi>)
  n87 = Bundle("Puff"=w113, "Puff Delay"=w112, "Puff Interval"=w111, "Puff Number"=w110, "Puff Stimulus Method"=w108) -> (w106:T4)  [unwired: 1 in]
  n88 = Bundle("Custom 2"=w23, "Custom 2 Delay"=w24, "Custom 2 Interval"=w25, "Custom 2 Number"=w26, "Custom 2 Stimulus Method"=w27) -> (w22:T5)  [unwired: 1 in]
  n89 = Bundle("Custom 1"=w96, "Custom 1 Delay"=w95, "Custom 1 Interval"=w94, "Custom 1 Number"=w93, "Custom 1 Stimulus Method"=w92) -> (w97:T6)  [unwired: 1 in]
  n90 = Bundle("Tap"=w117, "Tap Delay"=w116, "Tap Interval"=w115, "Tap Number"=w114, "Tap Stimulus Method"=w109) -> (w107:T7)  [unwired: 1 in]
  n91 = Bundle(w107, w106, w97, w22) -> (w10:T8)  [unwired: 1 in]
  n92 = Bundle("Run"=w105, "Set Region of Interest"=w119, "Clear Region of Interest"=w122, "Clear Reference Object(s)"=w121, "Set New Reference Object"=w120, "Advanced Settings"=w91) -> (w101:T9)  [unwired: 1 in]
  n93 = Bundle("Path"=w90, "Prefix"=w89, "Type of object to track"=w88, "Object Contrast (%)"=w87, "Fill Hysteresis (%)"=w86, "Maximum Object Size (pixels)"=w85, "Minimum Object Size (pixels)"=w84, "Object Size hysteresis (%)"=w83, "Image Binning"=w82, "Contour?"=w81, "Skeletonize?"=w80, "Frames of Adaptation"=w79, "Adaptation Rate"=w78, "Object Border"=w77, "Image Bit Depth"=w76, "Bit Depth from Camera?"=w75, "AFG resource name"=w74, "IMAQ Camera Interface Name"=w73, "Auto-start delay (s)"=w56, "Number of Image Adaptation Bands"=w55, "Experiment Duration (s)"=w54, "Tap"=w53, "Tap Delay"=w52, "Tap Interval"=w51, "Tap Number"=w50, "Tap Stimulus Method"=w49, "Advanced Tap Settings"=w48, "Puff"=w47, "Puff Delay"=w46, "Puff Interval"=w45, "Puff Number"=w44, "Puff Stimulus Method"=w43, "Advanced Puff Settings"=w42, "Custom 1"=w41, "Custom 1 Delay"=w40, "Custom 1 Interval"=w39, "Custom 1 Number"=w38, "Custom 1 Stimulus Method"=w37, "Advanced Custom 1 Settings"=w36, "puff fraction of time between is active"=w35, "time between puff onset"=w34, "tap fraction of time between is active"=w33, "time between tap onset"=w32, "Tap Train Number"=w31, "custom 1 fraction of time between is active"=w30, "time between custom 1 onset"=w29, "Custom 2"=w12, "Custom 2 Delay"=w13, "Custom 2 Interval"=w14, "Custom 2 Number"=w15, "Custom 2 Stimulus Method"=w16, "Advanced Custom 2 Settings"=w17, "custom 2 fraction of time between is active"=w18, "time between custom 2 onset"=w19, "Save"=w20, "Load"=w21, "Raw Image Save Interval (s)"=w11, "Turn on output aggregation?"=w9, "Turn on Background division algorithm"=w8, "Turn on external triggering of camera"=w6) -> (w102:T10)  [unwired: 1 in]
  n94 = Cluster To Array(cluster=w101) -> (array=w118:refnum<vi>[])
  n95 = call "make_buttons_available.vi"("array"=w118, "Make Available"=TRUE) -> ()
  n96 = call "make_controls_available.vi"("input cluster"=w102, "Make Available"=TRUE) -> ()
  n97 = Bundle(w10, w102, w101) -> (w100:T11)  [unwired: 1 in]
  n98 = flat-sequence {
    tunnel: [w125] -> w68
    tunnel: [w123] -> w67
    tunnel: w100 -> [w125]
    tunnel: [w207] -> w99
    tunnel: w68 -> [w207]
    tunnel: w67 -> [w195]
    tunnel: [w195] -> w66
    tunnel: w99 -> [w224]
    tunnel: [w224] -> w62
    tunnel: [w234] -> w60
    tunnel: w66 -> [w229]
    tunnel: [w228] -> w58
    tunnel: w62 -> [w378]
    tunnel: [w378] -> w61
    tunnel: w60 -> [w377]
    tunnel: [w377] -> w59
    tunnel: w58 -> [w376]
    tunnel: [w376] -> w57
    tunnel: [w373] -> w4
    tunnel: w61 -> [w426]
    tunnel: [w392] -> w98
    tunnel: w59 -> [w392]
    tunnel: [w426] -> w71
    tunnel: w57 -> [w420]
    tunnel: [w415] -> w65
    tunnel: [w399] -> w63
    tunnel: w4 -> [w384]
    tunnel: [w384] -> w3
    tunnel: w98 -> [w506]
    tunnel: [w479] -> w72
    tunnel: w71 -> [w479]
    tunnel: w65 -> [w472]
    tunnel: [w476] -> w64
    tunnel: w63 -> [w475]
    tunnel: w3 -> [w437]
    tunnel: [w437] -> w2
    tunnel: w72 -> [w804]
    tunnel: w64 -> [w802]
    tunnel: w2 -> [w799]
    frame #0 {
      n99 = property on="Query for Interface?" class="Bool (strict)"() -> ("Value"=w124:bool)  [unwired: 2 in, 2 out]
      n100 = case shown="False" w124 {
        tunnel: [w127 w154] -> w123
        frame False {
          n101 = property on="Image Data Input Source" class="Enum (strict)"() -> ("Value"=w129:T1)  [unwired: 2 in, 2 out]
          n102 = case shown="\"IMAQ interface\", Default" w129 {
            tunnel: [_ w141 _] -> w128
            tunnel: [w137 _ _] -> w131
            tunnel: [_ _ w150] -> w130
            frame "IMAQ interface", Default {
              n103 = property on="IMAQ Camera Interface Name" class="Str"() -> ("Value"=w134:string)  [unwired: 2 in, 2 out]
              n104 = call <vilib>:"IMAQ Init.vi"("Interface Name"=w134) -> ("error out"=w136:errorcluster, "IMAQ Session Out"=w135:refnum<k11>)  [unwired: 9 in]
              n105 = call <vilib>:"IMAQ Grab Setup.vi"("error in (no error)"=w136, "IMAQ Session In"=w135) -> ("error out"=w133:errorcluster, "IMAQ Session Out"=w137:refnum<k11>)  [unwired: 8 in]
              n106 = Unbundle(w133) -> ("status"=w132:bool)  [unwired: 2 out]
              n107 = case shown="True" w132 {
                frame False {
                }
                frame True {
                  n108 = flat-sequence {
                    frame #0 {
                      n109 = call "Display Message to User3"() -> ()  [unwired: 10 in, 2 out]
                    }
                    frame #1 {
                      n110 = property on="Query for Interface?" class="Bool (strict)"("Value"=TRUE ("Query for Interface?")) -> ()  [unwired: 2 in, 2 out]
                    }
                    frame #2 {
                      n111 = Stop(stop? (T)=TRUE) -> ()
                    }
                  }
                }
              }
            }
            frame "IMAQdx interface" {
              n112 = property on="IMAQdx camera interface name" class="IMAQdx (strict)"() -> ("Value"=w142:T2)  [unwired: 2 in, 2 out]
              n113 = call <vilib>:"IMAQdx Open Camera.vi"("Session In"=w142) -> ("error out"=w144:errorcluster, "Session Out"=w143:T2)  [unwired: 9 in]
              n114 = call <vilib>:"IMAQdx Configure Grab.vi"("error in"=w144, "Session In"=w143) -> ("error out"=w140:errorcluster, "Session Out"=w141:T2)  [unwired: 8 in]
              n115 = Unbundle(w140) -> ("status"=w145:bool)  [unwired: 2 out]
              n116 = case shown="True" w145 {
                frame False {
                }
                frame True {
                  n117 = flat-sequence {
                    frame #0 {
                      n118 = call "Display Message to User4"() -> ()  [unwired: 10 in, 2 out]
                    }
                    frame #1 {
                      n119 = property on="Query for Interface?" class="Bool (strict)"("Value"=TRUE ("Query for Interface?")) -> ()  [unwired: 2 in, 2 out]
                    }
                    frame #2 {
                      n120 = Stop(stop? (T)=TRUE) -> ()
                    }
                  }
                }
              }
            }
            frame "AVI file" {
              n121 = property on="AVI path" class="Path"() -> ("Value"=w151:path)  [unwired: 2 in, 2 out]
              n122 = call "IMAQ AVI Open"("AVI Path"=w151) -> ("error out"=w148:errorcluster, "Avi Refnum"=w150:T13)  [unwired: 9 in]
              n123 = Unbundle(w148) -> ("status"=w149:bool)  [unwired: 2 out]
              n124 = case shown="True" w149 {
                frame False {
                }
                frame True {
                  n125 = flat-sequence {
                    frame #0 {
                      n126 = call "Display Message to User5"() -> ()  [unwired: 10 in, 2 out]
                    }
                    frame #1 {
                      n127 = property on="Query for Interface?" class="Bool (strict)"("Value"=TRUE ("Query for Interface?")) -> ()  [unwired: 2 in, 2 out]
                    }
                    frame #2 {
                      n128 = Stop(stop? (T)=TRUE) -> ()
                    }
                  }
                }
              }
            }
          }
          n129 = property on="Turn on external triggering of camera" class="Bool (strict)"() -> ("Value"=w126:bool)  [unwired: 2 in, 2 out]
          n130 = Bundle("IMAQ Session Out"=w131, "Avi Refnum"=w130, "Value"=w129, "Session Out"=w128, "Value"=w126) -> (w127:T14)  [unwired: 1 in]
        }
        frame True {
          n131 = flat-sequence {
            tunnel: [w164] -> w161
            tunnel: [w170] -> w159
            tunnel: [w169] -> w157
            tunnel: [w168] -> w156
            tunnel: w161 -> [w176]
            tunnel: [w176] -> w160
            tunnel: w159 -> [w175]
            tunnel: [w175] -> w158
            tunnel: w157 -> [w174]
            tunnel: w156 -> [w173]
            tunnel: [w172] -> w155
            tunnel: w160 -> [w189]
            tunnel: w158 -> [_]
            tunnel: w155 -> [w188]
            tunnel: [w187] -> w154
            frame #0 {
              n132 = property on="IMAQ Camera Interface Name" class="Str"() -> ("Value"=w171:string)  [unwired: 2 in, 2 out]
              n133 = property on="Turn on external triggering of camera" class="Bool (strict)"() -> ("Value"=w162:bool)  [unwired: 2 in, 2 out]
              n134 = call "camera_selector.vi"("IMAQ interface name"=w171, "Use external trigger for camera control (IMAQ only)"=w162) -> ("output cluster"=w170:T15)
              n135 = Unbundle(w170) -> ("Value"=w167:refnum<k11>, "Value"=w166:refnum<k1>, "Value"=w165:T1, w164:T16, w169:bool, "Value"=w163:bool)
              n136 = Bundle("Value"=w167, "Value"=w166, "Value"=w165) -> (w168:T17)  [unwired: 1 in]
              n137 = property on="Turn on external triggering of camera" class="Bool (strict)"("Value"=w163) -> ()  [unwired: 2 in, 2 out]
            }
            frame #1 {
              n138 = case shown="False" w174 {
                tunnel: w173 -> [w177 _]
                tunnel: [w177 _] -> w172
                frame False {
                }
                frame True {
                  n139 = flat-sequence {
                    frame #0 {
                      n140 = call "Display Message to User2"() -> ()  [unwired: 10 in, 2 out]
                    }
                    frame #1 {
                      n141 = property on="Query for Interface?" class="Bool (strict)"("Value"=TRUE ("Query for Interface?")) -> ()  [unwired: 2 in, 2 out]
                    }
                    frame #2 {
                      n142 = Stop(stop? (T)=TRUE) -> ()
                    }
                  }
                }
              }
            }
            frame #2 {
              n143 = Unbundle(w189) -> ("Value"=w190:string, "Value"=w182:T2, "Value"=w181:path)
              n144 = Unbundle(w188) -> ("Value"=w186:refnum<k11>, "Value"=w185:refnum<k1>, "Value"=w183:T1)
              n145 = property on="IMAQ Camera Interface Name" class="Str"("Value"=w190) -> ()  [unwired: 2 in, 2 out]
              n146 = property on="IMAQdx camera interface name" class="IMAQdx (strict)"("Value"=w182) -> ()  [unwired: 2 in, 2 out]
              n147 = property on="AVI path" class="Path"("Value"=w181) -> ()  [unwired: 2 in, 2 out]
              n148 = property on="Turn on external triggering of camera" class="Bool (strict)"() -> ("Value"=w180:bool)  [unwired: 2 in, 2 out]
              n149 = Bundle("Value"=w186, "Value"=w185, "Value"=w183, "Value"=w182, "Value"=w180) -> (w187:T18)  [unwired: 1 in]
              n150 = property on="Query for Interface?" class="Bool (strict)"("Value"=FALSE ("Query for Interface?")) -> ()  [unwired: 2 in, 2 out]
              n151 = property on="Image Data Input Source" class="Enum (strict)"("Value"=w183) -> ()  [unwired: 2 in, 2 out]
            }
          }
        }
      }
    }
    frame #1 {
      w208 = T19 1 items=["Grayscale (U8)", "Grayscale (I16)", "Grayscale (SGL)", "Complex (CSG)", "RGB (U32)", "HSL (U32)", "RGB (U64)"] ("Image Type")
      # "MWT_getNewHandle"
      # "Create memory for displayed image"
      # "Dis/enable run button"
      # "Set initial state of important buttons"
      # "Initial Set up"
      n152 = disable-structure shown="Disabled" {
        frame Disabled {
          # "Stimulus Delivery Setup"
          n153 = call "Init_Stimulus.vi"() -> ()  [unwired: 1 in]
        }
        frame Enabled {
        }
      }
      n154 = property on="Stop" class="Bool (strict)"("Disabled"=u8 0, "Value"=FALSE) -> ()  [unwired: 2 in, 2 out]
      n155 = property on="Run" class="Bool (strict)"("Value"=FALSE) -> ()  [unwired: 2 in, 2 out]
      n156 = property on="Display/Don't Display" class="Bool (strict)"("Value"=TRUE) -> ()  [unwired: 2 in, 2 out]
      n157 = Unbundle(w207) -> (w193:T10)  [unwired: 2 out]
      n158 = property on="last acquired buffer" class="DigNum (strict)"("Value"=0 ("last acquired buffer")) -> ()  [unwired: 2 in, 2 out]
      n159 = local read "ROI Array"() -> (w214:dbl[][])
      n160 = call "init_ROI.vi"("Input ROI Array"=w214, "camera cluster"=w195) -> ("First Call? out"=w212:bool, "Output ROI Array"=w213:dbl[][])
      n161 = dll-call lib="C:/_WORKSPACE/DATA/PROJECTS/IMAQ/SOFTWARE/MWT NO STIM/MWT.dll" fn="MWT_getNewHandle"() -> ("return type"=w192:i32)  [unwired: 3 in, 2 out]
      "Tracker Handle" <- w192
      n162 = local write "First-call"(w212) -> ()
      n163 = call "set_in_library.vi"("Cluster"=w193, "camera cluster"=w195, "Tracker Handle"=w192, "Array"=w213) -> ("Directory Exists?"=w201:bool)  [unwired: 1 out]
      n164 = call "BitsPerPixel.vi"("camera cluster"=w195) -> ("BitsPerPixel"=w198:u32)
      n165 = call "GetWidthAndHeight.vi"("camera cluster"=w195) -> ("Width"=w197:u32, "Height"=w196:u32)
      n166 = local write "ROI Array"(w213) -> ()
      n167 = control-ref of="Directory Exists?"() -> (w200:refnum<vi>)
      n168 = call "IMAQ Create"("Image Name"="image data", "Image Type"=w208) -> ("New Image"=w211:T3, "error out"=w191:errorcluster)  [unwired: 3 in]
      n169 = Greater?(x=w198, y=u32 8) -> (0:w205:bool)
      n170 = Select(t=0, s=w201, f=2) -> (s? t:f=w202:i32)
      n171 = property on="Run" class="Bool (strict)"("Disabled"=w202) -> ()  [unwired: 2 in, 2 out]
      n172 = case shown="True" FALSE {
        tunnel: w205 -> [_ w219]
        frame False {
        }
        frame True {
          n173 = case shown="False" w219 {
            frame False {
              n174 = call "Display Message to User"() -> ()  [unwired: 10 in, 2 out]
            }
            frame True {
              # "Everything\nis fine."
            }
          }
        }
      }
      n175 = property class="Bool (strict)"(reference=w200, "Value"=w201) -> ()  [unwired: 1 in, 2 out]
      n176 = call "IMAQ SetImageSize"("error in (no error)"=w191, "Y Resolution"=w196, "X Resolution"=w197, "Image"=w211) -> ("Image Out"=w210:T3)  [unwired: 1 in, 1 out]
      n177 = property on="Image" class="ImageControl"("Value"=w210) -> ()  [unwired: 2 in, 2 out]
    }
    frame #2 {
      # "Initial feedback and settings configuration"
      # "Initial Constants with dummy values"
      n178 = local read "custom 1 timing array"() -> (w222:dbl[])
      n179 = local read "custom 2 timing array"() -> (w223:dbl[])
      n180 = local read "puff timing array"() -> (w221:dbl[])
      n181 = local read "tap timing array"() -> (w220:dbl[])
      n182 = local read "AFG resource name"() -> (w230:refnum<k15>)
      n183 = Unbundle(w224) -> (w225:T10)  [unwired: 2 out]
      n184 = call "get_tracker_settings.vi"("Cluster"=w225) -> ("settings value cluster"=w237:T20)
      n185 = while {
        shift-right: [w247] -> w235
        shift-left: w220 -> [w308]
        shift-right: [w311] -> _
        shift-left: T12 {"Value"=FALSE, "Value"=-1000.0, "Value"=-1000.0, "Value"=1000, "Value"=1000} ("output values cluster") -> [w280]
        shift-right: [w254] -> _
        shift-left: w237 -> [w314]
        shift-right: [w305] -> _
        shift-left: T12 {"Value"=FALSE, "Value"=-1000.0, "Value"=-1000.0, "Value"=1000, "Value"=1000} ("output values cluster") -> [w279]
        shift-right: [w246] -> w236
        shift-left: w221 -> [w307]
        shift-right: [w317] -> _
        shift-left: w230 -> [w318]
        tunnel: w224 -> [w301]
        shift-right: [w245] -> w232
        shift-left: w222 -> [w306]
        shift-right: [w304] -> _
        shift-left: T12 {"Value"=FALSE, "Value"=-1000.0, "Value"=-1000.0, "Value"=1000, "Value"=1000} ("output values cluster") -> [w278]
        shift-right: [w303] -> _
        shift-left: TRUE -> [w302]
        tunnel: w229 -> [w268]
        tunnel: [w268] -> w228
        shift-right: [w275] -> _
        shift-left: T12 {"Value"=FALSE, "Value"=-1000.0, "Value"=-1000.0, "Value"=1000, "Value"=1000} ("output values cluster") -> [w277]
        shift-right: [w244] -> w226
        shift-left: w223 -> [w276]
        stop <- w286 stop-if-true
        # "Note: Condition necessary\nbecause of potential discrepency\nbetween closing camera sessions\nand exiting the VI."
        # "Logic for \"begin after ... seconds\" function"
        # "Dis/enable run button"
        # "Feedback on setup stage"
        # "UI for ROIs"
        # "UI for advanced settings"
        # "UI for reference objects"
        # "Sets values in library,\nas well as saving and loading"
        # "Sets up the timing arrays \nfor the stimuli"
        # "Clean-up if stop is pressed."
        n186 = disable-structure shown="Disabled" {
          disable-tunnel: w318 -> [w325 _]
          disable-tunnel: [w324 _] -> w317
          disable-tunnel: [w321 _] -> w303
          disable-tunnel: w302 -> [w320 _]
          frame Disabled {
            # "AFG initialization"
            n187 = local read "AFG resource name"() -> (w326:refnum<k15>)
            n188 = Not Equal?(x=w326, y=w325) -> (x != y?=w323:bool)
            n189 = And(x=w323, y=w320) -> (x .and. y?=w322:bool)
            n190 = case shown="True" w322 {
              tunnel: [w328 w331] -> w324
              tunnel: w326 -> [_ w331]
              tunnel: w325 -> [w328 _]
              tunnel: [w327 FALSE] -> w321
              tunnel: w320 -> [w327 _]
              frame False {
              }
              frame True {
                n191 = call "AFG_Init.vi"("amplitude (1)"=1.0, "resource name"=w331, "frequency (1000000)"=100.0) -> ("instrument handle out"=w329:refnum<k15>)
                n192 = local write "AFG instrument handle"(w329) -> ()
              }
            }
          }
          frame Enabled {
          }
        }
        n193 = Unbundle(w301) -> (w281:T8, w270:T10)  [unwired: 1 out]
        n194 = Unbundle(w301) -> (w269:T9)  [unwired: 2 out]
        n195 = property on="User interface display slector" class="Ring (strict)"() -> ("Value"=w243:u16)  [unwired: 2 in, 2 out]
        n196 = case shown="0, Default" w243 {
          frame 0, Default {
            w334 = u16 0 items=["Raw Image", "Memory Image", "Fixed Image"] ("What to display")
            n197 = property on="Display/Don't Display" class="Bool (strict)"("Value"=TRUE ("Display/Don't Display")) -> ()  [unwired: 2 in, 2 out]
            n198 = property on="What to display" class="Ring (strict)"("Value"=w334) -> ()  [unwired: 2 in, 2 out]
          }
          frame 1 {
            w336 = u16 1 items=["Raw Image", "Memory Image", "Fixed Image"] ("What to display")
            n199 = property on="Display/Don't Display" class="Bool (strict)"("Value"=TRUE ("Display/Don't Display")) -> ()  [unwired: 2 in, 2 out]
            n200 = property on="What to display" class="Ring (strict)"("Value"=w336) -> ()  [unwired: 2 in, 2 out]
          }
          frame 2 {
            w338 = u16 2 items=["Raw Image", "Memory Image", "Fixed Image"] ("What to display")
            n201 = property on="Display/Don't Display" class="Bool (strict)"("Value"=TRUE ("Display/Don't Display")) -> ()  [unwired: 2 in, 2 out]
            n202 = property on="What to display" class="Ring (strict)"("Value"=w338) -> ()  [unwired: 2 in, 2 out]
          }
          frame 3 {
            w340 = u16 2 items=["Raw Image", "Memory Image", "Fixed Image"] ("What to display")
            n203 = property on="Display/Don't Display" class="Bool (strict)"("Value"=FALSE ("Display/Don't Display")) -> ()  [unwired: 2 in, 2 out]
            n204 = property on="What to display" class="Ring (strict)"("Value"=w340) -> ()  [unwired: 2 in, 2 out]
          }
        }
        n205 = local read "AFG Settings"() -> (w309:dbl[][])
        n206 = local read "Image Bit Depth"() -> (w264:u32)
        n207 = property on="Tracker Handle" class="DigNum (strict)"() -> ("Value"=w316:i32)  [unwired: 2 in, 2 out]
        n208 = property on="last acquired buffer" class="DigNum (strict)"() -> ("Value"=w292:i32)  [unwired: 2 in, 2 out]
        n209 = Bundle("AFG Settings"=w309, "tap timing array"=w308, "puff timing array"=w307, "custom timing array"=w306, "custom 2 timing array"=w276, w281, w270, "output values cluster"=w280, "output values cluster"=w279, "output values cluster"=w278, "output values cluster"=w277) -> (w310:T21)  [unwired: 1 in]
        n210 = Bundle(w268, "Value"=w316, "Value"=w292) -> (w313:T22)  [unwired: 1 in]
        n211 = call "all_things_stimulus.vi"("input cluster"=w310) -> ("output cluster"=w312:T23)
        n212 = Bundle(w313, w269, "Image Bit Depth"=w264) -> (w242:T24)  [unwired: 1 in]
        n213 = Unbundle(w312) -> ("output values cluster"=w311:T25, "Output Array"=w251:dbl[], "output values cluster"=w305:T25, "Output Array"=w250:dbl[], "output values cluster"=w304:T25, "Output Array"=w249:dbl[], "AFG Settings"=w256:dbl[][], "output values cluster"=w275:T25, "Output Array"=w248:dbl[])
        n214 = call "set_or_clear_reference_object.vi"("input cluster"=w242) -> ("last acquired buffer out"=w294:i32)
        n215 = local read "ROI Array"() -> (w315:dbl[][])
        n216 = property on="last acquired buffer" class="DigNum (strict)"("Value"=w294) -> ()  [unwired: 2 in, 2 out]
        n217 = control-ref of="Directory Exists?"() -> (w255:refnum<vi>)
        n218 = Unbundle(w301) -> (w267:T10)  [unwired: 2 out]
        n219 = Bundle(w313, w270, "ROI Array"=w315, "settings value cluster"=w314, "AFG Settings"=w256, "Output Array"=w251, "Output Array"=w250, "Output Array"=w249, "Output Array"=w248) -> (w241:T26)  [unwired: 1 in]
        n220 = call "Tracker_Settings.vi"("input cluster"=w241, "Directory Exists?"=w255) -> ("output cluster"=w257:T27)
        n221 = Bundle(w267, w268) -> (w300:T28)  [unwired: 1 in]
        n222 = Unbundle(w257) -> ("Output  ROI Array"=w253:dbl[][], "settings value cluster"=w254:T20, "AFG Settings"=w252:dbl[][], "tap timing array"=w247:dbl[], "puff timing array"=w246:dbl[], "custom timing array"=w245:dbl[], "custom 2 timing array"=w244:dbl[])
        n223 = property on="last acquired buffer" class="DigNum (strict)"() -> ("Value"=w289:i32)  [unwired: 2 in, 2 out]
        n224 = property on="Tracker Handle" class="DigNum (strict)"() -> ("Value"=w288:i32)  [unwired: 2 in, 2 out]
        n225 = property on="Stop" class="Bool (strict)"() -> ("Value"=w271:bool)  [unwired: 2 in, 2 out]
        n226 = property on="Advanced Settings" class="Bool (strict)"() -> ("Value"=w299:bool)  [unwired: 2 in, 2 out]
        n227 = property on="Display/Don't Display" class="Bool (strict)"() -> ("Value"=w273:bool)  [unwired: 2 in, 2 out]
        n228 = Not(x=w271) -> (.not. x?=w274:bool)
        n229 = Bundle(w268, "Value"=w288, "Value"=w289) -> (w287:T22)  [unwired: 1 in]
        n230 = case shown="True" w299 {
          tunnel: w300 -> [_ w349]
          frame False {
          }
          frame True {
            n231 = call "advanced_settings.vi"("input cluster"=w349) -> ("Output AFG resource name"=w351:refnum<k15>)  [unwired: 1 out]
            n232 = local write "AFG resource name"(w351) -> ()
            n233 = property on="Advanced Settings" class="Bool (strict)"("Value"=FALSE ("Advanced Settings")) -> ()  [unwired: 2 in, 2 out]
          }
        }
        n234 = And(x=w273, y=w274) -> (x .and. y?=w272:bool)
        n235 = local write "AFG Settings"(w252) -> ()
        n236 = case shown="True" w272 {
          tunnel: w287 -> [_ w370]
          frame False {
          }
          frame True {
            n237 = local read "Image Binning"() -> (w369:u16)
            n238 = property on="What to display" class="Ring (strict)"() -> ("Value"=w365:u16)  [unwired: 2 in, 2 out]
            n239 = Bundle(w370, "Image Binning"=w369, "Value"=w365) -> (w358:T29)  [unwired: 1 in]
            n240 = call "initial_feedback.vi"("input cluster"=w358) -> ("output cluster"=w371:T30)
            n241 = Unbundle(w371) -> ("Acquired Buffer Number"=w368:i32, "return type"=w367:i32, "destination"=w366:i16[][])
            n242 = local read "Image Bit Depth"() -> (w360:u32)
            n243 = local read "Image"() -> (w372:T3)
            n244 = local write "Objects Found"(w367) -> ()
            n245 = property on="last acquired buffer" class="DigNum (strict)"("Value"=w368) -> ()  [unwired: 2 in, 2 out]
            n246 = call "IMAQ ArrayToImage"("Image Pixels (I16)"=w366, "Image"=w372) -> ("error out"=w359:errorcluster, "Image Out"=w364:T3)  [unwired: 8 in]
            n247 = call "IMAQ Image Bit Depth"("Image"=w364, "Bit Depth (0)"=w360, "error in (no error)"=w359, "Get/Set Bit Depth? (Set)"=TRUE) -> ("Image Out"=w363:T3, "error out"=→"error out":errorcluster)  [unwired: 9 in, 1 out]
            n248 = local write "Image"(w363) -> ()
          }
        }
        n249 = local write "ROI Array"(w253) -> ()
        n250 = local write "custom 2 timing array"(w244) -> ()
        n251 = local write "custom 1 timing array"(w245) -> ()
        n252 = local write "puff timing array"(w246) -> ()
        n253 = local write "tap timing array"(w247) -> ()
        n254 = local read "ROI Array"() -> (w261:dbl[][])
        n255 = Unbundle(w301) -> (w266:T10, w265:T9)  [unwired: 1 out]
        n256 = property on="First-call" class="Bool (strict)"() -> ("Value"=w262:bool)  [unwired: 2 in, 2 out]
        n257 = property on="Auto-start delay (s)" class="DigNum (strict)"() -> ("Value"=w283:i32)  [unwired: 2 in, 2 out]
        n258 = Greater Than 0?(x=w283) -> (x > 0?=w282:bool)
        n259 = control-ref of="Directory Exists?"() -> (w290:refnum<vi>)
        n260 = property on="last acquired buffer" class="DigNum (strict)"() -> ("Value"=w263:i32)  [unwired: 2 in, 2 out]
        n261 = property on="Tracker Handle" class="DigNum (strict)"() -> ("Value"=w291:i32)  [unwired: 2 in, 2 out]
        n262 = Bundle(w268, "Value"=w291, "Value"=w263) -> (w293:T22)  [unwired: 1 in]
        n263 = case shown="True" w282 {
          tunnel: [FALSE w348] -> w284
          frame False {
          }
          frame True {
            n264 = property on="Run" class="Bool (strict)"() -> ("Disabled"=w344:u8)  [unwired: 2 in, 2 out]
            n265 = Not Equal To 0?(x=w344) -> (x != 0?=w343:bool)
            n266 = property on="Auto-start delay (s)" class="DigNum (strict)"() -> ("Value"=w347:i32)  [unwired: 2 in, 2 out]
            n267 = call "Elapsed Time"("Time Target (s)"=w347, "Reset"=w343) -> ("Elapsed Time (s)"=w346:dbl, "Time has Elapsed"=w348:bool)  [unwired: 10 in, 6 out]
            n268 = Subtract(x=w347, y=w346) -> (x-y=w345:dbl)
            n269 = property on="Auto-start in (s)" class="DigNum (strict)"("Value"=w345) -> ()  [unwired: 2 in, 2 out]
          }
        }
        n270 = Bundle(w293, "ROI Array"=w261, "Value"=w262, w266, w265, "Directory Exists?"=w290) -> (w240:T31)  [unwired: 1 in]
        n271 = call "ROI.vi"("input cluster"=w240) -> ("Acquired Buffer Number"=w258:u32, "Output First-call"=w259:bool, "Output ROI Array"=w260:dbl[][])
        n272 = property on="Stop" class="Bool (strict)"() -> ("Value"=w319:bool)  [unwired: 2 in, 2 out]
        n273 = property on="First-call" class="Bool (strict)"("Value"=w259) -> ()  [unwired: 2 in, 2 out]
        n274 = local write "ROI Array"(w260) -> ()
        n275 = property on="last acquired buffer" class="DigNum (strict)"("Value"=w258) -> ()  [unwired: 2 in, 2 out]
        n276 = case shown="True" w319 {
          tunnel: w268 -> [_ w352]
          frame False {
          }
          frame True {
            n277 = flat-sequence {
              tunnel: w352 -> [w355]
              frame #0 {
                # "MWT_killHandle"
                n278 = property on="Tracker Handle" class="DigNum (strict)"() -> ("Value"=w354:i32)  [unwired: 2 in, 2 out]
                n279 = dll-call lib="C:/_WORKSPACE/DATA/PROJECTS/IMAQ/SOFTWARE/MWT NO STIM/MWT.dll" fn="MWT_killHandle"("handle"=w354) -> ()  [unwired: 5 in, 2 out]
                n280 = Bundle(w355, 0) -> (w353:T32)  [unwired: 1 in]
                n281 = call "camera_closer.vi"("input cluster"=w353) -> ()
              }
              frame #1 {
                n282 = Stop(stop? (T)=TRUE) -> ()
              }
            }
          }
        }
        n283 = property on="Directory Exists?" class="Bool (strict)"() -> ("Value"=w295:bool)  [unwired: 2 in, 2 out]
        n284 = property on="Run" class="Bool (strict)"() -> ("Value"=w285:bool)  [unwired: 2 in, 2 out]
        n285 = Select(t=0, s=w295, f=2) -> (s? t:f=w296:i32)
        n286 = Or(x=w285, y=w284) -> (x .or. y?=w286:bool)
        n287 = property on="Run" class="Bool (strict)"("Disabled"=w296) -> ()  [unwired: 2 in, 2 out]
      }
      n288 = Bundle("tap timing array"=w235, "puff timing array"=w236, "custom timing array"=w232, "custom 2 timing array"=w226) -> (w234:T33)  [unwired: 1 in]
    }
    frame #3 {
      # "Save value of display selector for later restoration."
      # "Special case for AVI input: Setting initial frame."
      n289 = Unbundle(w376) -> ("Avi Refnum"=w375:T13, "Value"=w374:T1)  [unwired: 3 out]
      n290 = case shown="\"IMAQ interface\"" w374 {
        tunnel: w375 -> [w383 _ _]
        frame "AVI file" {
          # "In the case of AVIs,\nreset the AVI frame\nto the \"beginning\" for\nprocessing."
          n291 = call "IMAQ AVI Get Info"("Avi Refnum"=w383) -> ("Frame Data"=w382:T34)  [unwired: 6 in, 4 out]
          n292 = Unbundle(w382) -> ("framesPerSecond"=w381:u32)  [unwired: 4 out]
          n293 = property on="Auto-start delay (s)" class="DigNum (strict)"() -> ("Value"=w380:i32)  [unwired: 2 in, 2 out]
          n294 = Multiply(x=w381, y=w380) -> (x*y=w379:u32)
          n295 = property on="last acquired buffer" class="DigNum (strict)"("Value"=w379) -> ()  [unwired: 2 in, 2 out]
        }
        frame "IMAQdx interface" {
          # "Do nothing for this interface"
        }
        frame "IMAQ interface" {
          # "Do nothing for this interface"
        }
      }
      n296 = property on="User interface display slector" class="Ring (strict)"() -> ("Value"=w373:u16)  [unwired: 2 in, 2 out]
    }
    frame #4 {
      w385 = u16 3 items=["Raw Image", "Memory Image", "Fixed Image", "Nothing", ""] ("User interface display slector")
      w424 = FALSE ("Make Available")
      # "Output setup and disabling of controls"
      n297 = disable-structure shown="Disabled" {
        frame Disabled {
          w432 = 0
          # "Configure initial settings of AFG."
          n298 = local read "AFG Settings"() -> (w429:dbl[][])
          n299 = Index Array(array=w429, index (row) #1=w432, index (col) #1=1, index (row) #2=w432, index (col) #2=2) -> (element #1=w431:dbl, element #2=w430:dbl)
          n300 = local read "AFG instrument handle"() -> (w435:refnum<k15>)
          n301 = call "AFG_Waveform_settings.vi"("amplitude (1)"=w430, "frequency (1000000)"=w431, "instrument handle"=w435) -> ()
        }
        frame Enabled {
        }
      }
      n302 = property on="Image Binning" class="Ring (strict)"() -> ("Value"=w421:u16)  [unwired: 2 in, 2 out]
      n303 = property on="Frames of Adaptation" class="DigNum (strict)"() -> ("Value"=w422:i32)  [unwired: 2 in, 2 out]
      n304 = property on="User interface display slector" class="Ring (strict)"("Value"=w385) -> ()  [unwired: 2 in, 2 out]
      n305 = property on="Stop" class="Bool (strict)"("Disabled"=u8 0) -> ()  [unwired: 2 in, 2 out]
      n306 = property on="Display/Don't Display" class="Bool (strict)"("Value"=FALSE) -> ()  [unwired: 2 in, 2 out]
      n307 = Unbundle(w426) -> (w394:T10, w402:T9)  [unwired: 1 out]
      n308 = property on="Tracker Handle" class="DigNum (strict)"() -> ("Value"=w423:i32)  [unwired: 2 in, 2 out]
      n309 = property on="Prefix" class="Str"() -> ("Value"=w400:string)  [unwired: 2 in, 2 out]
      n310 = property on="last acquired buffer" class="DigNum (strict)"() -> ("Value"=w419:i32)  [unwired: 2 in, 2 out]
      n311 = local read "AFG Settings"() -> (w393:dbl[][])
      n312 = Concatenate Strings(w400, ".set") -> (w398:string)
      n313 = local read "Image"() -> (w414:T3)
      n314 = local read "ROI Array"() -> (w396:dbl[][])
      n315 = Cluster To Array(cluster=w402) -> (array=w425:refnum<vi>[])
      n316 = Bundle(w420, "Value"=w419) -> (w418:T35)  [unwired: 1 in]
      n317 = call "make_buttons_available.vi"("array"=w425, "Make Available"=w424) -> ()
      n318 = call "make_controls_available.vi"("input cluster"=w394, "Make Available"=w424) -> ()
      n319 = Unbundle(w418) -> (w417:T36)  [unwired: 1 out]
      n320 = Bundle(w418, "Value"=w423, "Value"=w422, "Value"=w421, "Image"=w414) -> (w387:T37)  [unwired: 1 in]
      n321 = Unbundle(w392) -> ("tap timing array"=w390:dbl[], "puff timing array"=w391:dbl[], "custom timing array"=w389:dbl[], "custom 2 timing array"=w388:dbl[])
      n322 = call "set_date_and_create_initial_memory_image.vi"("input cluster"=w387) -> ("Acquired Buffer Number"=w406:u32, "sub_directory"=w403:string)
      n323 = property on="Path" class="Path"() -> ("Value"=w404:path)  [unwired: 2 in, 2 out]
      n324 = Bundle(w417, "Acquired Buffer Number"=w406) -> (w386:T38)  [unwired: 1 in]
      n325 = property on="Prefix" class="Str"() -> ("Value"=w408:string)  [unwired: 2 in, 2 out]
      n326 = Build Path(base path=w404, name or relative path=w403) -> (appended path=w399:path)
      n327 = Build Path(base path=w399, name or relative path=w398) -> (appended path=w395:path)
      n328 = Bundle(w394, "appended path"=w395, "ROI Array"=w396, "AFG Settings"=w393, "tap timing array"=w390, "puff timing array"=w391, "custom timing array"=w389, "custom 2 timing array"=w388) -> (w397:T39)  [unwired: 1 in]
      n329 = call "save_configuration.vi"("input cluster"=w397) -> ()
      n330 = Unbundle(w386) -> (w416:T36)  [unwired: 1 out]
      n331 = call "smart_get.vi"("Input Image"=w414, "Cluster"=w386) -> ("Image Out"=w413:T3, "Acquired Buffer Number"=w405:i32)
      n332 = Concatenate Strings(w408, ".png") -> (w411:string)
      n333 = Bundle(w416, "Acquired Buffer Number"=w405) -> (w415:T40)  [unwired: 1 in]
      n334 = Build Path(base path=w399, name or relative path=w411) -> (appended path=w410:path)
      n335 = property on="last acquired buffer" class="DigNum (strict)"("Value"=w405) -> ()  [unwired: 2 in, 2 out]
      n336 = call-poly "IMAQ Write File 2"("Use bit depth? (false)"=TRUE, "Image Quality"=u32 750, "File Path"=w410, "Image"=w413) -> ()  [unwired: 6 in, 2 out]
    }
    frame #5 {
      # "MWT_reportImageCorrectionAlgorithm"
      # "Individual Frame Saving and AFG control\nNOTE: These functions do not make sense when an AVI is used as input, and so are disabled in that case."
      # "Processing"
      n337 = Unbundle(w472) -> (w471:T36)  [unwired: 1 out]
      n338 = Unbundle(w471) -> ("Value"=w438:T1)  [unwired: 4 out]
      n339 = Not Equal?(x=w438, y=T1."AVI file" ("Image Data Input Source")) -> (x != y?=w473:bool)
      n340 = Unbundle(w506) -> ("tap timing array"=w445:dbl[], "puff timing array"=w443:dbl[], "custom timing array"=w441:dbl[], "custom 2 timing array"=w439:dbl[])
      n341 = case shown="True" w473 {
        tunnel: w475 -> [_ w533]
        tunnel: w472 -> [_ w530]
        frame False {
        }
        frame True {
          # "AFG control"
          n342 = local read "Image"() -> (w534:T3)
          n343 = property on="Raw Image Save Interval (s)" class="DigNum (strict)"() -> ("Value"=w529:dbl)  [unwired: 2 in, 2 out]
          n344 = call "IMAQ Create"("Image Name"="more_garbage") -> ("New Image"=w537:T3)  [unwired: 4 in, 1 out]
          n345 = Greater Than 0?(x=w529) -> (x > 0?=w535:bool)
          n346 = call "IMAQ Copy"("Image Dst"=w537, "Image Src"=w534) -> ("Image Dst Out"=w538:T3)  [unwired: 4 in, 1 out]
          n347 = Multiply(x=w529, y=1000.0) -> (x*y=w531:dbl)
          n348 = case shown="True" w535 {
            tunnel: w533 -> [_ w549]
            tunnel: w531 -> [_ w547]
            tunnel: w538 -> [_ w548]
            tunnel: w530 -> [_ w544]
            frame False {
            }
            frame True {
              n349 = call "get_time.vi"("input cluster"=w544) -> ("millisecond timer value"=w545:u32)
              n350 = while {
                tunnel: w549 -> [w567]
                tunnel: w547 -> [w560]
                tunnel: w548 -> [w566]
                tunnel: w544 -> [w551]
                shift-right: [w562] -> _
                shift-left: 0 -> [w561]
                shift-right: [w559] -> _
                shift-left: w545 -> [w564]
                tunnel: w545 -> [w558]
                stop <- w550 stop-if-true
                # "Larval-specific addition"
                n351 = Unbundle(w551) -> (w554:T36)  [unwired: 1 out]
                n352 = call "get_time.vi"("input cluster"=w551) -> ("millisecond timer value"=w559:u32)
                n353 = property on="last acquired buffer" class="DigNum (strict)"() -> ("Value"=w553:i32)  [unwired: 2 in, 2 out]
                n354 = Bundle(w554, "Value"=w553) -> (w552:T35)  [unwired: 1 in]
                n355 = Subtract(x=w559, y=w558) -> (x-y=w556:u32)
                n356 = call "elapsed_time.vi"("Time since last update"=w561, "Initial Time"=w564, "Current Time"=w559) -> ("Elapsed Time"=w557:i32)
                n357 = call "smart_get.vi"("Input Image"=w566, "Cluster"=w552) -> ("Image Out"=w565:T3, "Acquired Buffer Number"=w555:i32)
                n358 = Greater?(x=w557, y=w560) -> (0:w563:bool)
                n359 = property on="last acquired buffer" class="DigNum (strict)"("Value"=w555) -> ()  [unwired: 2 in, 2 out]
                n360 = case shown="True" w563 {
                  tunnel: w565 -> [_ w580]
                  tunnel: w567 -> [_ w579]
                  tunnel: [w568 0] -> w562
                  tunnel: w557 -> [w568 _]
                  tunnel: w556 -> [_ w569]
                  frame False {
                  }
                  frame True {
                    n361 = Format Into String(format string="%05d", w569) -> (resulting string=w576:string)  [unwired: 2 in, 1 out]
                    n362 = property on="Prefix" class="Str"() -> ("Value"=w577:string)  [unwired: 2 in, 2 out]
                    n363 = Concatenate Strings(w577, w576, ".png") -> (w574:string)
                    n364 = Build Path(base path=w579, name or relative path=w574) -> (appended path=w573:path)
                    n365 = call-poly "IMAQ Write File 2"("Use bit depth? (false)"=TRUE, "Image Quality"=u32 750, "File Path"=w573, "Image"=w580) -> ()  [unwired: 6 in, 2 out]
                  }
                }
                n366 = property on="Proccessing loop stopped?" class="Bool (strict)"() -> ("Value"=w550:bool)  [unwired: 2 in, 2 out]
              }
            }
          }
          n367 = local read "AFG Settings"() -> (w542:dbl[][])
          n368 = Array Size(array=w542) -> (size(s)=w543:i32[])
          n369 = call "get_time.vi"("input cluster"=w530) -> ("millisecond timer value"=w539:u32)
          n370 = Index Array(array=w543) -> (element=w540:i32)  [unwired: 1 in]
          n371 = while {
            tunnel: w542 -> [w589]
            shift-right: [w587] -> _
            shift-left: 0 -> [w588]
            tunnel: w540 -> [w591]
            tunnel: w539 -> [w590]
            tunnel: w530 -> [w582]
            stop <- w584 continue-if-true
            n372 = call "get_time.vi"("input cluster"=w582) -> ("millisecond timer value"=w586:u32)
            n373 = Less?(x=w588, y=w591) -> (x < y?=w585:bool)
            n374 = case shown="True" w585 {
              tunnel: w586 -> [_ w595]
              tunnel: w590 -> [_ w596]
              tunnel: w589 -> [_ w599]
              tunnel: w588 -> [w592 w598]
              tunnel: [w592 w597] -> w587
              frame False {
              }
              frame True {
                n375 = Index Array(array=w599, index (row) #1=w598, index (col) #1=0 ("disabled index (col)"), index (row) #2=w598, index (col) #2=1, index (row) #3=w598, index (col) #3=2) -> (element #1=w593:dbl, element #2=w604:dbl, element #3=w605:dbl)
                n376 = Subtract(x=w595, y=w596) -> (x-y=w594:u32)
                n377 = Greater Or Equal?(x=w594, y=w593) -> (x >= y?=w601:bool)
                n378 = disable-structure shown="Disabled" {
                  disable-tunnel: w605 -> [w610 _]
                  disable-tunnel: w604 -> [w609 _]
                  disable-tunnel: w601 -> [w608 _]
                  disable-tunnel: w598 -> [w607 _]
                  disable-tunnel: [w606 _] -> w597
                  frame Disabled {
                    n379 = case shown="True" w608 {
                      tunnel: w609 -> [_ w613]
                      tunnel: w610 -> [_ w612]
                      tunnel: w607 -> [w611 w616]
                      tunnel: [w611 w615] -> w606
                      frame False {
                      }
                      frame True {
                        n380 = local read "AFG instrument handle"() -> (w614:refnum<k15>)
                        n381 = Increment(x=w616) -> (x+1=w615:i32)
                        n382 = call "AFG_Waveform_settings.vi"("amplitude (1)"=w612, "frequency (1000000)"=w613, "instrument handle"=w614) -> ()
                      }
                    }
                  }
                  frame Enabled {
                  }
                }
              }
            }
            n383 = property on="Proccessing loop stopped?" class="Bool (strict)"() -> ("Value"=w581:bool)  [unwired: 2 in, 2 out]
            n384 = Not(x=w581) -> (.not. x?=w583:bool)
            n385 = And(x=w583, y=w585) -> (x .and. y?=w584:bool)
          }
        }
      }
      n386 = control-ref of="XY Graph"() -> (w492:refnum<vi>)
      n387 = control-ref of="XY Graph 2"() -> (w491:refnum<vi>)
      n388 = control-ref of="XY Graph 3"() -> (w490:refnum<vi>)
      n389 = control-ref of="XY Graph 4"() -> (w489:refnum<vi>)
      n390 = local read "Image"() -> (w507:T3)
      n391 = control-ref of="Graph Input"() -> (w496:refnum<vi>)
      n392 = control-ref of="Graph Input 2"() -> (w495:refnum<vi>)
      n393 = control-ref of="Graph Input 3"() -> (w494:refnum<vi>)
      n394 = control-ref of="Graph Input 4"() -> (w493:refnum<vi>)
      n395 = property on="tap fraction of time between is active" class="Arr (strict)"() -> ("Value"=w503:sgl[][])  [unwired: 2 in, 2 out]
      n396 = property on="time between tap onset" class="Arr (strict)"() -> ("Value"=w502:i32[][])  [unwired: 2 in, 2 out]
      n397 = property on="Tap Train Number" class="Arr (strict)"() -> ("Value"=w501:i32[][])  [unwired: 2 in, 2 out]
      n398 = call "IMAQ GetImageSize"("Image"=w507) -> ("Y Resolution"=w511:i32, "X Resolution"=w510:i32)  [unwired: 3 in, 1 out]
      n399 = property on="Image Binning" class="Ring (strict)"() -> ("Value"=w461:u16)  [unwired: 2 in, 2 out]
      n400 = Bundle("Graph Input"=w496, "Graph Input 2"=w495, "Graph Input 3"=w494, "Graph Input 4"=w493, "XY Graph"=w492, "XY Graph 2"=w491, "XY Graph 3"=w490, "XY Graph 4"=w489) -> (w488:T41)  [unwired: 1 in]
      n401 = property on="puff fraction of time between is active" class="Arr (strict)"() -> ("Value"=w499:sgl[][])  [unwired: 2 in, 2 out]
      n402 = property on="time between puff onset" class="Arr (strict)"() -> ("Value"=w498:i32[][])  [unwired: 2 in, 2 out]
      n403 = property on="Tracker Handle" class="DigNum (strict)"() -> ("Value"=w447:i32)  [unwired: 2 in, 2 out]
      n404 = property on="custom 2 fraction of time between is active" class="Arr (strict)"() -> ("Value"=w466:sgl[][])  [unwired: 2 in, 2 out]
      n405 = property on="time between custom 2 onset" class="Arr (strict)"() -> ("Value"=w465:i32[][])  [unwired: 2 in, 2 out]
      n406 = property on="custom 1 fraction of time between is active" class="Arr (strict)"() -> ("Value"=w486:sgl[][])  [unwired: 2 in, 2 out]
      n407 = property on="time between custom 1 onset" class="Arr (strict)"() -> ("Value"=w487:i32[][])  [unwired: 2 in, 2 out]
      n408 = call "get_time.vi"("input cluster"=w472) -> ("millisecond timer value"=w474:u32)
      n409 = Divide(x=w511, y=w461) -> (x/y=w515:dbl)
      n410 = Divide(x=w510, y=w461) -> (x/y=w516:dbl)
      n411 = dll-call lib="C:/_WORKSPACE/DATA/PROJECTS/IMAQ/SOFTWARE/MWT NO STIM/MWT.dll" fn="MWT_reportImageCorrectionAlgorithm"("handle"=w447) -> ("return type"=w449:i32)  [unwired: 4 in, 2 out]
      n412 = Bundle("Value"=w503, "Value"=w502, "Value"=w501) -> (w500:T42)  [unwired: 1 in]
      n413 = local read "Image"() -> (w508:T3)
      n414 = property on="Tap" class="Bool (strict)"() -> ("Value"=w482:bool)  [unwired: 2 in, 2 out]
      n415 = Round To Nearest(number=w515) -> (nearest integer value=w517:dbl)
      n416 = Round To Nearest(number=w516) -> (nearest integer value=w518:dbl)
      n417 = Array Size(array=w443) -> (size(s)=w444:i32)
      n418 = Array Size(array=w439) -> (size(s)=w440:i32)
      n419 = Array Size(array=w441) -> (size(s)=w442:i32)
      n420 = Greater Than 0?(x=w449) -> (x > 0?=w448:bool)
      n421 = Array Size(array=w445) -> (size(s)=w446:i32)
      n422 = Bundle("Value"=w499, "Value"=w498) -> (w497:cluster{"Value":sgl[][], "Value":i32[][]})  [unwired: 1 in]
      n423 = Bundle("Value"=w466, "Value"=w465) -> (w467:cluster{"Value":sgl[][], "Value":i32[][]})  [unwired: 1 in]
      n424 = Bundle("Value"=w486, "Value"=w487) -> (w485:cluster{"Value":sgl[][], "Value":i32[][]})  [unwired: 1 in]
      n425 = call "IMAQ Create"("Image Name"="display") -> ("New Image"=w523:T3)  [unwired: 4 in, 1 out]
      n426 = To Long Integer(number=w517) -> (32bit integer=w513:i32)
      n427 = To Long Integer(number=w518) -> (32bit integer=w512:i32)
      n428 = case shown="True" w448 {
        tunnel: [i32[] [] w526] -> w450
        frame False {
        }
        frame True {
          n429 = Initialize Array(-1 ("element"), 200 ("dimension size")) -> (w526:i32[])
        }
      }
      n430 = call "IMAQ Copy"("Image Dst"=w523, "Image Src"=w508) -> ("Image Dst Out"=w460:T3)  [unwired: 4 in, 1 out]
      n431 = property on="Puff" class="Bool (strict)"() -> ("Value"=w481:bool)  [unwired: 2 in, 2 out]
      n432 = Initialize Array(i16 0 ("element"), w513, w512) -> (w509:i16[][])
      n433 = property on="Custom 2" class="Bool (strict)"() -> ("Value"=w469:bool)  [unwired: 2 in, 2 out]
      n434 = property on="Custom 1" class="Bool (strict)"() -> ("Value"=w480:bool)  [unwired: 2 in, 2 out]
      n435 = call "Init_Data_array.vi"() -> ("Data Cluster"=w519:T43)
      n436 = call "IMAQ GetImageSize"("Image"=w460) -> ("Y Resolution"=w463:i32, "X Resolution"=w462:i32)  [unwired: 3 in, 1 out]
      n437 = while {
        tunnel: w508 -> [w688]
        shift-right: [w654] -> _
        shift-left: w474 -> [w692]
        tunnel: w445 -> [w740]
        shift-right: [w735] -> _
        shift-left: 0 -> [w739]
        tunnel: w482 -> [w737]
        tunnel: w446 -> [w738]
        tunnel: w474 -> [w693]
        shift-right: [w742] -> _
        shift-left: 0 -> [w736]
        shift-right: [w714] -> _
        shift-left: 0 -> [w694]
        shift-right: [w713] -> _
        shift-left: w519 -> [w719]
        tunnel: w444 -> [w731]
        shift-right: [w725] -> _
        shift-left: 0 -> [w727]
        tunnel: w481 -> [w730]
        shift-right: [w724] -> _
        shift-left: 0 -> [w729]
        tunnel: w443 -> [w732]
        tunnel: w500 -> [w651]
        tunnel: w497 -> [w642]
        tunnel: w488 -> [w717]
        tunnel: w485 -> [w640]
        shift-right: [w703] -> _
        shift-left: 0 -> [w711]
        shift-right: [w702] -> _
        shift-left: 0 -> [w708]
        tunnel: w442 -> [w710]
        tunnel: w480 -> [w709]
        tunnel: w441 -> [w712]
        shift-right: [w701] -> _
        shift-left: 1 -> [w687]
        shift-right: [w696] -> _
        shift-left: 0 -> [w700]
        shift-right: [w695] -> _
        shift-left: w509 -> [w695]
        shift-right: [w684] -> w476
        shift-left: w472 -> [w682]
        tunnel: w467 -> [w634]
        shift-right: [w674] -> _
        shift-left: 0 -> [w678]
        shift-right: [w675] -> _
        shift-left: 0 -> [w681]
        tunnel: w440 -> [w679]
        tunnel: w469 -> [w680]
        tunnel: w439 -> [w669]
        tunnel: w463 -> [w659]
        tunnel: w462 -> [w658]
        tunnel: w460 -> [w657]
        shift-right: [w649] -> _
        shift-left: 0 -> [w653]
        shift-right: [w648] -> _
        shift-left: 0 -> [w652]
        shift-right: [w645] -> _
        shift-left: 0 -> [w647]
        shift-right: [w644] -> _
        shift-left: 0 -> [w646]
        shift-right: [w637] -> _
        shift-left: 0 -> [w639]
        shift-right: [w636] -> _
        shift-left: 0 -> [w638]
        shift-right: [w631] -> _
        shift-left: 0 -> [w633]
        shift-right: [w630] -> _
        shift-left: 0 -> [w632]
        shift-right: [w628] -> _
        shift-left: 0 -> [w629]
        shift-right: [w626] -> _
        shift-left: w450 -> [w627]
        stop <- w621 stop-if-true
        # "Elapsed time\nCurrent time\ntime since last frame"
        # "Event is a bitmask"
        # "Mark Stimulus event"
        # "Retrieve statisical data in to the graphs"
        # "Run the actual experiment."
        n438 = call "get_time.vi"("input cluster"=w682) -> ("millisecond timer value"=w654:u32)
        n439 = Subtract(x=w654, y=w693) -> (x-y=w625:u32)
        n440 = Divide(x=w625, y=sgl 1000.0) -> (x/y=w666:sgl)
        n441 = property on="User interface display slector" class="Ring (strict)"() -> ("Value"=w620:u16)  [unwired: 2 in, 2 out]
        n442 = call "GetStimulusArrayValues.vi"("tap train index"=w629, "time between onset index"=w652, "fraction of time between index"=w653, "Cluster"=w651, "time since beginning of run"=w625) -> ("tap train index out"=w628:i32, "time between onset index out"=w648:i32, "fraction of time between index out"=w649:i32, "stimulus settings"=w650:cluster{"outy3":sgl, "outy3":i32, "Value":i32})
        n443 = call "GetOtherStimulusArrayValues.vi"("time between onset index"=w638, "fraction of time between index"=w639, "Cluster"=w640, "time since beginning of run"=w625) -> ("time between onset index out"=w636:i32, "fraction of time between index out"=w637:i32, "stimulus settings"=w641:cluster{"outy3":sgl, "outy3":i32})
        n444 = call "GetOtherStimulusArrayValues.vi"("time between onset index"=w632, "fraction of time between index"=w633, "Cluster"=w634, "time since beginning of run"=w625) -> ("time between onset index out"=w630:i32, "fraction of time between index out"=w631:i32, "stimulus settings"=w635:cluster{"outy3":sgl, "outy3":i32})
        n445 = call "GetOtherStimulusArrayValues.vi"("time between onset index"=w646, "fraction of time between index"=w647, "Cluster"=w642, "time since beginning of run"=w625) -> ("time between onset index out"=w644:i32, "fraction of time between index out"=w645:i32, "stimulus settings"=w643:cluster{"outy3":sgl, "outy3":i32})
        n446 = case shown="0, Default" w620 {
          frame 0, Default {
            w760 = u16 0 items=["Raw Image", "Memory Image", "Fixed Image"] ("What to display")
            n447 = property on="Display/Don't Display" class="Bool (strict)"("Value"=TRUE ("Display/Don't Display")) -> ()  [unwired: 2 in, 2 out]
            n448 = property on="What to display" class="Ring (strict)"("Value"=w760) -> ()  [unwired: 2 in, 2 out]
          }
          frame 1 {
            w762 = u16 1 items=["Raw Image", "Memory Image", "Fixed Image"] ("What to display")
            n449 = property on="Display/Don't Display" class="Bool (strict)"("Value"=TRUE ("Display/Don't Display")) -> ()  [unwired: 2 in, 2 out]
            n450 = property on="What to display" class="Ring (strict)"("Value"=w762) -> ()  [unwired: 2 in, 2 out]
          }
          frame 2 {
            w764 = u16 2 items=["Raw Image", "Memory Image", "Fixed Image"] ("What to display")
            n451 = property on="Display/Don't Display" class="Bool (strict)"("Value"=TRUE ("Display/Don't Display")) -> ()  [unwired: 2 in, 2 out]
            n452 = property on="What to display" class="Ring (strict)"("Value"=w764) -> ()  [unwired: 2 in, 2 out]
          }
          frame 3 {
            w766 = u16 2 items=["Raw Image", "Memory Image", "Fixed Image"] ("What to display")
            n453 = property on="Display/Don't Display" class="Bool (strict)"("Value"=FALSE ("Display/Don't Display")) -> ()  [unwired: 2 in, 2 out]
            n454 = property on="What to display" class="Ring (strict)"("Value"=w766) -> ()  [unwired: 2 in, 2 out]
          }
        }
        n455 = call "elapsed_time.vi"("Time since last update"=w700, "Initial Time"=w692, "Current Time"=w654) -> ("Elapsed Time"=w697:i32)
        n456 = Bundle("custom timing array"=w712, w711, w710, "Value"=w709, w708, "stimulus settings"=w641) -> (w707:T44)  [unwired: 1 in]
        n457 = Bundle("custom 2 timing array"=w669, w678, w679, "Value"=w680, w681, "stimulus settings"=w635) -> (w671:T45)  [unwired: 1 in]
        n458 = property on="Minimum time between events(ms)" class="DigNum (strict)"() -> ("Value"=w624:u32)  [unwired: 2 in, 2 out]
        n459 = Unbundle(w682) -> (w686:T36)  [unwired: 1 out]
        n460 = property on="last acquired buffer" class="DigNum (strict)"() -> ("Value"=w685:i32)  [unwired: 2 in, 2 out]
        n461 = Bundle("puff timing array"=w732, w727, w731, "Value"=w730, w729, "stimulus settings"=w643) -> (w733:T46)  [unwired: 1 in]
        n462 = control-ref of="Time until Next Puff"() -> (w734:refnum<vi>)
        n463 = control-ref of="Time until Next Custom 2"() -> (w672:refnum<vi>)
        n464 = control-ref of="Time until Next Custom 1"() -> (w706:refnum<vi>)
        n465 = Bundle(w686, "Value"=w685) -> (w684:T35)  [unwired: 1 in]
        n466 = property on="Display/Don't Display" class="Bool (strict)"() -> ("Value"=w660:bool)  [unwired: 2 in, 2 out]
        n467 = control-ref of="Time until Next Tap"() -> (w745:refnum<vi>)
        n468 = property on="Seconds into Experiment" class="DigNum (strict)"("Value"=w666) -> ()  [unwired: 2 in, 2 out]
        n469 = Bundle("tap timing array"=w740, w739, w738, "Value"=w737, w736, "stimulus settings"=w650) -> (w741:T47)  [unwired: 1 in]
        n470 = Bundle(w625, "millisecond timer value"=w654, "millisecond timer value"=w692, "Value"=w624) -> (w673:T48)  [unwired: 1 in]
        n471 = call "smart_get.vi"("Input Image"=w688, "Cluster"=w684) -> ("Image Out"=w662:T3, "Acquired Buffer Number"=w683:i32)
        n472 = property on="Tracker Handle" class="DigNum (strict)"() -> ("Value"=w718:i32)  [unwired: 2 in, 2 out]
        n473 = case shown="True" w660 {
          tunnel: [i16[][] [] ("Image Pixels (I16)") w775] -> w661
          tunnel: w659 -> [_ w772]
          tunnel: w658 -> [_ w771]
          frame False {
          }
          frame True {
            n474 = property on="Image Binning" class="Ring (strict)"() -> ("Value"=w770:u16)  [unwired: 2 in, 2 out]
            n475 = Divide(x=w772, y=w770) -> (x/y=w777:dbl)
            n476 = Divide(x=w771, y=w770) -> (x/y=w778:dbl)
            n477 = Round To Nearest(number=w777) -> (nearest integer value=w779:dbl)
            n478 = Round To Nearest(number=w778) -> (nearest integer value=w780:dbl)
            n479 = To Long Integer(number=w779) -> (32bit integer=w774:i32)
            n480 = To Long Integer(number=w780) -> (32bit integer=w773:i32)
            n481 = Initialize Array(i16 0 ("element"), w774, w773) -> (w775:i16[][])
          }
        }
        n482 = Greater?(x=w697, y=1000) -> (0:w699:bool)
        n483 = Bundle(w673, "Time until Next Tap"=w745, w741) -> (w744:T49)  [unwired: 1 in]
        n484 = Bundle(w673, "Time until Next Puff"=w734, w733) -> (w726:T50)  [unwired: 1 in]
        n485 = Bundle(w673, "Time until Next Custom 1"=w706, w707) -> (w705:T51)  [unwired: 1 in]
        n486 = Bundle(w673, "Time until Next Custom 2"=w672, w671) -> (w670:T52)  [unwired: 1 in]
        n487 = property on="Seconds into Experiment" class="DigNum (strict)"() -> ("Value"=w617:dbl)  [unwired: 2 in, 2 out]
        n488 = property on="Experiment Duration (s)" class="DigNum (strict)"() -> ("Value"=w618:dbl)  [unwired: 2 in, 2 out]
        n489 = Bundle("millisecond timer value"=w654, "millisecond timer value"=w692, w694, w666, "Data Cluster"=w719, "Value"=w718, w717) -> (w716:T53)  [unwired: 1 in]
        n490 = disable-structure shown="Disabled" {
          disable-tunnel: w744 -> [w756 _]
          disable-tunnel: [w755 _] -> w743
          disable-tunnel: [w754 _] -> w728
          disable-tunnel: w726 -> [w753 _]
          disable-tunnel: w705 -> [w752 _]
          disable-tunnel: [w751 _] -> w704
          disable-tunnel: [w750 _] -> w677
          disable-tunnel: w670 -> [w749 _]
          frame Disabled {
            # "Custom 1 Stimuli"
            # "Custom 2 Stimuli"
            # "Puff Stimuli"
            # "Tap stimuli"
            n491 = call "puff_stimulus_generator.vi"("input cluster"=w753) -> ("output cluster"=w754:cluster{i32, i32, "Elapsed Time":i32})
            n492 = call "custom_1_stimulus_generator.vi"("input cluster"=w752) -> ("output cluster"=w751:cluster{i32, i32, "Elapsed Time":i32})
            n493 = call "custom_2_stimulus_generator.vi"("input cluster"=w749) -> ("output cluster"=w750:cluster{i32, i32, "Elapsed Time":i32})
            n494 = call "tap_stimulus_generator.vi"("input cluster"=w756) -> ("output cluster"=w755:T54)
          }
          frame Enabled {
          }
        }
        n495 = property on="last acquired buffer" class="DigNum (strict)"("Value"=w683) -> ()  [unwired: 2 in, 2 out]
        n496 = case shown="True" w699 {
          tunnel: w687 -> [w782 w786]
          tunnel: [w781 1] -> w701
          tunnel: w697 -> [w783 w789]
          tunnel: [w783 0] -> w696
          frame False {
            n497 = Increment(x=w782) -> (x+1=w781:i32)
          }
          frame True {
            n498 = Divide(x=1000 ("y"), y=w789) -> (x/y=w787:dbl)
            n499 = Divide(x=w787, y=w786) -> (x/y=→"seconds per frame":dbl)
          }
        }
        n500 = Greater Than 0?(x=w618) -> (x > 0?=w619:bool)
        n501 = Unbundle(w728) -> (w690:i32, w725:i32, "Elapsed Time"=w724:i32)
        "# Puffs Delivered" <- w725
        n502 = Unbundle(w704) -> (w689:i32, w703:i32, "Elapsed Time"=w702:i32)
        "# Custom 1's Delivered" <- w703
        n503 = Unbundle(w677) -> (w676:i32, w674:i32, "Elapsed Time"=w675:i32)
        "# Custom 2's Delivered" <- w674
        n504 = call "graph_data_acquisition_and_display.vi"("input cluster"=w716) -> ("output cluster"=w715:T55)
        n505 = Unbundle(w743) -> (w691:i32, "Tap Number"=w735:i32, "Elapsed Time"=w742:i32)
        "# Taps Delivered" <- w735
        n506 = case shown="True" w619 {
          tunnel: w618 -> [_ w758]
          tunnel: w617 -> [_ w757]
          frame False {
          }
          frame True {
            n507 = Subtract(x=w758, y=w757) -> (x-y=w759:dbl)
            n508 = property on="Auto-end in (s)" class="DigNum (strict)"("Value"=w759) -> ()  [unwired: 2 in, 2 out]
          }
        }
        n509 = property on="Tracker Handle" class="DigNum (strict)"() -> ("Value"=w668:i32)  [unwired: 2 in, 2 out]
        n510 = property on="Image Binning" class="Ring (strict)"() -> ("Value"=w667:u16)  [unwired: 2 in, 2 out]
        n511 = property on="What to display" class="Ring (strict)"() -> ("Value"=w665:u16)  [unwired: 2 in, 2 out]
        n512 = property on="Display/Don't Display" class="Bool (strict)"() -> ("Value"=w663:bool)  [unwired: 2 in, 2 out]
        n513 = property on="Image Bit Depth" class="DigNum (strict)"() -> ("Value"=w664:u32)  [unwired: 2 in, 2 out]
        n514 = Unbundle(w715) -> ("Elapsed Time"=w714:i32, "Data Cluster"=w713:T43)
        n515 = formula code="int32 event = 0b0;\nif( e1 > 0 ) \n  event += 0b0001;\nif( e2 > 0 ) \n  event += 0b0010;\nif( e3 > 0 )\n  event += 0b0100;\nif( e4 > 0 )\n  event += 0b1000;"("e1"=w691, "e2"=w690, "e3"=w689, "e4"=w676) -> ("event"=w656:i32)
        n516 = Greater Or Equal?(x=w617, y=w618) -> (x >= y?=w622:bool)
        n517 = Greater Than 0?(x=w618) -> (x > 0?=w623:bool)
        n518 = And(x=w622, y=w623) -> (x .and. y?=w746:bool)
        n519 = property on="Stop" class="Bool (strict)"() -> ("Value"=w747:bool)  [unwired: 2 in, 2 out]
        n520 = Bundle(w656, "Value"=w668, "Value"=w667, w666, "Value"=w665, "Value"=w663, "Value"=w664, "Image Out"=w662, "Image Pixels (I16)"=w661, w627) -> (w655:T56)  [unwired: 1 in]
        n521 = Or(x=w746, y=w747) -> (x .or. y?=w621:bool)
        n522 = property on="Proccessing loop stopped?" class="Bool (strict)"("Value"=w621) -> ()  [unwired: 2 in, 2 out]
        n523 = call "processing_steps.vi"("input cluster"=w655) -> ("output cluster"=w723:T57)
        n524 = Unbundle(w723) -> ("return value"=w722:i32, "return value"=→"error count":i32, "Image Pixels (I16) out"=w720:i16[][], "coordinates"=w626:i32[])
        n525 = case shown="True" w621 {
          frame False {
          }
          frame True {
            n526 = property on="Stop" class="Bool (strict)"("Value"=TRUE ("Stop")) -> ()  [unwired: 2 in, 2 out]
          }
        }
        n527 = case shown="True" w663 {
          tunnel: w720 -> [_ w798]
          tunnel: w657 -> [_ w793]
          frame False {
          }
          frame True {
            n528 = property on="Image Bit Depth" class="DigNum (strict)"() -> ("Value"=w795:u32)  [unwired: 2 in, 2 out]
            n529 = call "IMAQ ArrayToImage"("Image Pixels (I16)"=w798, "Image"=w793) -> ("error out"=w791:errorcluster, "Image Out"=w797:T3)  [unwired: 8 in]
            n530 = call "IMAQ Image Bit Depth"("Image"=w797, "Bit Depth (0)"=w795, "error in (no error)"=w791, "Get/Set Bit Depth? (Set)"=TRUE) -> ("Image Out"=w796:T3, "error out"=→"error out 2":errorcluster)  [unwired: 9 in, 1 out]
            n531 = local write "Image"(w796) -> ()
          }
        }
        n532 = property on="Objects Found" class="DigNum (strict)"("Value"=w722) -> ()  [unwired: 2 in, 2 out]
      }
      "Go" <- TRUE ("Go")
    }
    frame #6 {
      w803 = TRUE ("Make Available")
      # "Restore value of display selector."
      # "Finalization, including cleanup and \nrestoration of initial control state."
      # "MWT_complete"
      # "MWT_killHandle"
      n533 = property on="User interface display slector" class="Ring (strict)"("Value"=w799) -> ()  [unwired: 2 in, 2 out]
      n534 = property on="Tracker Handle" class="DigNum (strict)"() -> ("Value"=w806:i32)  [unwired: 2 in, 2 out]
      n535 = call "camera_closer.vi"("input cluster"=w802) -> ()
      n536 = Unbundle(w804) -> (w801:T10, w800:T9)  [unwired: 1 out]
      n537 = dll-call lib="C:/_WORKSPACE/DATA/PROJECTS/IMAQ/SOFTWARE/MWT NO STIM/MWT.dll" fn="MWT_complete"("handle"=w806) -> ("handle"=w807:i32)  [unwired: 4 in, 2 out]
      n538 = Cluster To Array(cluster=w800) -> (array=w805:refnum<vi>[])
      n539 = call "make_buttons_available.vi"("array"=w805, "Make Available"=w803) -> ()
      n540 = dll-call lib="C:/_WORKSPACE/DATA/PROJECTS/IMAQ/SOFTWARE/MWT NO STIM/MWT.dll" fn="MWT_killHandle"("handle"=w807) -> ()  [unwired: 5 in, 2 out]
      n541 = call "make_controls_available.vi"("input cluster"=w801, "Make Available"=w803) -> ()
    }
  }
  n542 = flat-sequence {
    tunnel: [w808] -> w1
    tunnel: w1 -> [w825]
    frame #0 {
      # "Synchronization using DAQ"
      n543 = local write "Go"(FALSE ("Go")) -> ()
      n544 = property on="Stop" class="Bool (strict)"("Value"=FALSE ("Stop")) -> ()  [unwired: 2 in, 2 out]
      n545 = call <vilib>:"Application Directory.vi"() -> ("Application Directory"=w810:path)
      n546 = Build Path(base path=w810, name or relative path="Config.ini") -> (appended path=w814:path)
      n547 = Wait (ms)(milliseconds to wait=u32 100) -> ()  [unwired: 1 out]
      n548 = call <vilib>:"Open Config Data.vi"("configuration file path"=w814) -> ("refnum"=w818:T58)  [unwired: 8 in, 2 out]
      n549 = call-poly <vilib>:"Read Key.vi"("section"="PARAM", "default value"="Dev1/port2/line0", "key"="DAQ ID", "refnum"=w818) -> ("error out"=w811:errorcluster, "value"=w812:string, "refnum out"=w815:T58)  [unwired: 4 in, 1 out]
      n550 = call <vilib>:"Close Config Data.vi"("error in (no error)"=w811, "refnum"=w815) -> ()  [unwired: 8 in, 2 out]
      n551 = call-poly <vilib>:"DAQmx Create Virtual Channel.vi"("lines"=w812, "error in"=w811) -> ("task out"=w808:refnum<k21>)  [unwired: 12 in, 1 out]
    }
    frame #1 {
      n552 = while {
        tunnel: w825 -> [w827]
        tunnel: [w826] -> w824
        stop <- w829 stop-if-true
        # "Synchronization"
        n553 = local read "Go"() -> (w828:bool)
        n554 = property on="Stop" class="Bool (strict)"() -> ("Value"=w829:bool)  [unwired: 2 in, 2 out]
        n555 = Wait (ms)(milliseconds to wait=u32 100) -> ()  [unwired: 1 out]
        n556 = call-poly <vilib>:"DAQmx Write.vi"("task/channels in"=w827, "data"=w828) -> ("task out"=w826:refnum<k21>)  [unwired: 11 in, 2 out]
      }
      n557 = call-poly <vilib>:"DAQmx Write.vi"("task/channels in"=w824, "data"=FALSE) -> ("task out"=w823:refnum<k21>)  [unwired: 11 in, 2 out]
      n558 = call <vilib>:"DAQmx Stop Task.vi"("task/channels in"=w823) -> ()  [unwired: 13 in, 2 out]
    }
  }
  n559 = flat-sequence {
    frame #0 {
      # "Synchronization via TCP/IP"
      n560 = local write "Go"(FALSE ("Go")) -> ()
      n561 = property on="Stop" class="Bool (strict)"("Value"=FALSE ("Stop")) -> ()  [unwired: 2 in, 2 out]
      n562 = Wait (ms)(milliseconds to wait=u32 100) -> ()  [unwired: 1 out]
    }
    frame #1 {
      n563 = while {
        stop <- w834 stop-if-true
        # "Synchronization"
        n564 = property on="Stop" class="Bool (strict)"() -> ("Value"=w834:bool)  [unwired: 2 in, 2 out]
        n565 = TCP Open Connection(remote port or service name=u16 1000 ("port")) -> (connection ID=w838:refnum<k5>, error out=w836:errorcluster)  [unwired: 4 in]
        n566 = Wait (ms)(milliseconds to wait=u32 100) -> ()  [unwired: 1 out]
        n567 = case shown="No Error" w836 {
          tunnel: w838 -> [w846 _]
          frame No Error {
            n568 = while {
              shift-right: [w854] -> w845
              shift-left: w846 -> [w855]
              tunnel: [w848] -> w841
              stop <- w853 stop-if-true
              n569 = Wait (ms)(milliseconds to wait=u32 100) -> ()  [unwired: 1 out]
              n570 = local read "Go"() -> (w850:bool)
              n571 = case shown="True" w850 {
                tunnel: ["0" ("Cmd") "1" ("Cmd")] -> w851
                frame False {
                }
                frame True {
                }
              }
              n572 = property on="Stop" class="Bool (strict)"() -> ("Value"=w847:bool)  [unwired: 2 in, 2 out]
              n573 = TCP Write(connection ID=w855, data in=w851, 9:100 ("timeout ms (25000)")) -> (connection ID out=w854:refnum<k5>, error out=w848:errorcluster)  [unwired: 1 in, 1 out]
              n574 = Or(x=w848, y=w847) -> (x .or. y?=w853:bool)
            }
            n575 = TCP Write(connection ID=w845, data in="0", error in (no error)=w841, 9:100 ("timeout ms (25000)")) -> (connection ID out=w843:refnum<k5>, error out=w842:errorcluster)  [unwired: 1 out]
            n576 = TCP Close Connection(connection ID=w843, error in (no error)=w842) -> (error out=w844:errorcluster)  [unwired: 1 in, 1 out]
            n577 = call <vilib>:"Clear Errors.vi"("error in (no error)"=w844) -> ()  [unwired: 5 in, 2 out]
          }
          frame Error {
          }
        }
      }
    }
  }
  "Objects Found" <- w28
  "Seconds into Experiment" <- w28
  "Time until Next Puff" <- w28
  "Time until Next Tap" <- w28
  "First-call" <- TRUE ("First-call")
  "Proccessing loop stopped?" <- FALSE ("Proccessing loop stopped?")
  "Image" <- T3 refnum ("Image")
  "XY Graph" <- w7
  "XY Graph 2" <- w7
  "XY Graph 3" <- w7
  "XY Graph 4" <- w7
  "Time until Next Custom 1" <- w28
  "Auto-start in (s)" <- w28
  "Time until Next Custom 2" <- w28
